vi "WS1050 36 DUT Reliability HD_Cycling Ver1.5a.vi"() -> ()   [LabVIEW 2012]
uses:
  WS_VCAP Driver 029/Source/WSVCAP Shell/Type Defs/WSVCAP SHL I2C DUT Mask Mode Enum.ctl
  <vilib>/Utility/file.llb/Read From Spreadsheet File (DBL).vi
panel:
  out "VISA resource name out":refnum<visa-resource-name>="GPIB0::3::INSTR"
  out "error out 2":errorcluster={"status"=TRUE, "code"=-63192, "source"="niLvFpga_Open_PXI-7813R.vi"}
  in  "Reg1_Bit Cntrl":string[](array[string])=["01", "02", "04", "08", "10", "20", "40", "80", "03", "06", "0C", "D8", "33", "66", "CC", "07", "0E", "1C", "38", "70", "E0", "0F", "1E", "3C", "78", "F0", "1F", "3E", "7C", "F8", "3F", "7E", "FC", "7F", "FE", "FD", "FB", "F7", "EF", "DF", "BF", "7F", "FC", "F9", "F3", "E7", "CF", "9F", "3F", "F8", "F1", "E3", "C7", "8F", "1F", "F0", "E1", "C3", "87", "0F", "E0", "C1", "83", "07", "C0", "81", "03", "AA", "55", "00"]
  out "date string":string="5/19/2014"
  out "PS1 Out":refnum<visa-resource-name>
  out "Ke2000 Out":refnum<visa-resource-name>="GPIB0::9::INSTR"
  in  "VPI_Cmd":string[](array[string])=["00", "3B", "00"]
  in  "VPI Name":string[](array[string])=["All_Drivers OFF", "All Drivers ON", "All Drivers OFF2"]
  in  "Tab Control":T1(tab)
  in  "Board#":string="BRD5"
  in  "Serial Number":string[][](table)=[["DUT", "SN"], ["DUT1", "1"], ["DUT2", "2"], ["DUT3", "3"], ["DUT4", "4"], ["DUT5", "5"], ["DUT6", "6"], ["DUT7", "7"], ["DUT8", "8"], ["DUT9", "9"], ["DUT10", "10"], ["DUT11", "11"], ["DUT12", "12"], ["DUT13", "13"], ["DUT14", "14"], ["DUT15", "15"], ["DUT16", "16"], ["DUT17", "17"], ["DUT18", "18"], ["DUT19", "19"], ["DUT20", "20"], ["DUT21", "21"], ["DUT22", "22"], ["DUT23", "23"], ["DUT24", "24"], ["DUT25", "25"], ["DUT26", "26"], ["DUT27", "27"], ["DUT28", "28"], ["DUT29", "29"], ["DUT30", "30"], ["DUT31", "31"], ["DUT32", "32"], ["DUT33", "33"], ["DUT34", "34"], ["DUT35", "35"], ["DUT36", "36"]]
  in  "Wafer#":string="T7-EB"
  in  "File Name":string="CYC_WS1050_T7_EB_65C_40V_25DC_EMPTY_BRD5_151017_1"
  in  "TMN DC\\CAP Data Log File Path":path=path "C:/WS1050 36 DUT Data"
  in  "Test Program":string="WS1050 36 DUT Reliability HD_Cycling Ver1.5a"
  in  "Comment":string="CYC65C40V"
  in  "Calibration":bool
  out "AR  Measurent(Hz)":dbl
  in  "PS1 Source":refnum<visa-resource-name>="GPIB0::5::INSTR"
  in  "Ke2000":refnum<visa-resource-name>="GPIB0::9::INSTR"
  out "Simulate FPGA":bool
  out "Online":bool
  out "AR Cycling(Hz)":dbl=5000000.0
  in  "Ke2400":refnum<visa-resource-name>="GPIB0::3::INSTR"
  in  "Initialize AD7747":bool
  in  "DUT Mask Mode":T2=enum."All"
  in  "RFFE Slave Address":u8=7 caption="Slave Address" format="0x%02x"
  out "Activity Log":string="05/19/2014 -- 12:24:35.853::WSVCAP::APP::Application Started\n05/19/2014 -- 12:24:37.606::WSVCAP::WSVCAP SHL::WR I2C-REG:0x0A;MASK:0xFFFFFFFFFFFF;C1 DATA:22:22:22:22:22:22:22:22:22:22:22:22:22:22:22:22;C2 DATA:22:22:22:22:22:22:22:22:22:22:22:22:22:22:22:22;C3 DATA:22:22:22:22:22:22:22:22:22:22:22:22:22:22:22:22\r\n05/19/2014 -- 12:24:37.773::WSVCAP::WSVCAP SHL::WR I2C-ST:0,0,4,1\r\n05/19/2014 -- 12:24:37.903::WSVCAP::WSVCAP SHL::RD I2C-BYTES:4;ADD:0x00;MASK:0xFFFFFFFFFFFF\r\n05/19/2014 -- 12:24:38.045::WSVCAP::WSVCAP SHL::RD I2C:C1 DATA:2:2:2:2:2:2:2:2:2:2:2:2:2:2:2:2|A7:A9:AA:82:82:7F:82:81:82:81:83:82:81:82:82:81|46:36:BB:88:44:A3:E9:2B:32:20:ED:25:BB:3D:68:B|2C:6A:EB:A7:22:56:FE:CC:36:82:D7:B0:3B:48:F9:CC;C2 DATA:2:2:2:2:2:2:2:2:2:2:2:2:2:2:2:2|94:94:94:80:80:80:80:80:81:7E:7E:81:80:7E:80:80|47:33:15:82:62:B:E8:1C:D7:C3:7D:41:7C:B7:4C:2A|C4:B4:AE:8:1E:D1:4E:37:11:C0:6F:63:42:9D:63:B5;C3 DATA:2:2:2:2:2:2:2:2:2:2:2:2:2:2:2:2|95:95:95:81:81:7E:81:80:84:7D:80:83:81:7E:7F:80|AB:C4:14:B5:7B:52:DF:C9:79:5D:5F:30:99:31:1E:F4|6E:5C:F7:A8:C3:EB:7B:EF:33:92:89:77:4D:67:75:DD;STATUS:0:0:4:0\r\n05/19/2014 -- 12:24:38.046::WSVCAP::WSVCAP SHL::WR I2C-REG:0x0A;MASK:0xFFFFFFFFFFFF;C1 DATA:22:22:22:22:22:22:22:22:22:22:22:22:22:22:22:22;C2 DATA:22:22:22:22:22:22:22:22:22:22:22:22:22:22:22:22;C3 DATA:22:22:22:22:22:22:22:22:22:22:22:22:22:22:22:22\r\n05/19/2014 -- 12:24:38.089::WSVCAP::WSVCAP SHL::WR I2C-ST:0,0,4,1\r\n05/19/2014 -- 12:24:38.219::WSVCAP::WSVCAP SHL::RD I2C-BYTES:4;ADD:0x00;MASK:0xFFFFFFFFFFFF\r\n05/19/2014 -- 12:24:38.362::WSVCAP::WSVCAP SHL::RD I2C:C1 DATA:2:2:2:2:2:2:2:2:2:2:2:2:2:2:2:2|A7:AB:AA:82:82:82:83:83:82:82:82:82:7F:82:82:81|4B:32:96:83:3E:61:43:17:25:62:AB:4D:A2:40:2E:5|3C:76:2B:B4:EE:E4:A9:1A:AA:A:26:C7:21:2E:87:5B;C2 DATA:2:2:2:2:2:2:2:2:2:2:2:2:2:2:2:2|94:94:94:80:80:80:80:80:80:7F:80:81:80:80:7F:80|4A:32:19:7D:19:6C:79:46:61:7F:4B:B8:A5:30:F3:14|B4:70:A:8C:9C:DC:43:FA:1E:A:C6:21:A:A9:13:F3;C3 DATA:2:2:2:2:2:2:2:2:2:2:2:2:2:2:2:2|95:97:94:81:80:81:82:81:80:7E:81:84:7F:81:80:80|B2:32:D0:A7:9E:4C:AB:D4:EE:D9:F0:82:B7:91:7:FF|C1:91:B6:3D:D8:E:1B:4F:9F:6A:F1:6C:E7:3F:7:BA;STATUS:0:0:4:0\r\n05/19/2014 -- 12:24:38.364::WSVCAP::WSVCAP SHL::WR I2C-REG:0x0A;MASK:0xFFFFFFFFFFFF;C1 DATA:22:22:22:22:22:22:22:22:22:22:22:22:22:22:22:22;C2 DATA:22:22:22:22:22:22:22:22:22:22:22:22:22:22:22:22;C3 DATA:22:22:22:22:22:22:22:22:22:22:22:22:22:22:22:22\r\n05/19/2014 -- 12:24:38.406::WSVCAP::WSVCAP SHL::WR I2C-ST:0,0,4,1\r\n05/19/2014 -- 12:24:38.536::WSVCAP::WSVCAP SHL::RD I2C-BYTES:4;ADD:0x00;MASK:0xFFFFFFFFFFFF\r\n05/19/2014 -- 12:24:38.678::WSVCAP::WSVCAP SHL::RD I2C:C1 DATA:2:2:2:2:2:2:2:2:2:2:2:2:2:2:2:2|A7:A9:AB:82:82:81:82:82:82:82:82:82:82:82:82:81|46:71:4C:87:43:3D:7F:FC:25:4F:8E:54:97:3E:60:8C|AA:F4:1F:B5:CE:43:1F:36:9:87:9C:78:86:5:B6:8E;C2 DATA:2:2:2:2:2:2:2:2:2:2:2:2:2:2:2:2|94:94:94:80:7F:7F:80:80:80:80:80:81:80:80:80:80|49:36:18:7D:6E:C5:E4:3C:81:2E:41:D3:75:71:E3:72|E8:D3:E6:D1:E0:48:AE:D4:54:D:E8:8E:B4:41:68:4;C3 DATA:2:2:2:2:2:2:2:2:2:2:2:2:2:2:2:2|95:95:95:81:7F:7F:81:81:81:81:81:84:81:81:82:81|B3:F5:90:AB:82:69:7B:93:D0:77:E8:D5:E8:8C:84:E8|B9:AC:EE:2B:B6:71:8F:4A:74:31:56:BB:8A:B7:A0:C8;STATUS:0:0:4:0\r\n05/19/2014 -- 12:24:38.681::WSVCAP::WSVCAP SHL::WR I2C-REG:0x0A;MASK:0xFFFFFFFFFFFF;C1 DATA:22:22:22:22:22:22:22:22:22:22:22:22:22:22:22:22;C2 DATA:22:22:22:22:22:22:22:22:22:22:22:22:22:22:22:22;C3 DATA:22:22:22:22:22:22:22:22:22:22:22:22:22:22:22:22\r\n05/19/2014 -- 12:24:38.723::WSVCAP::WSVCAP SHL::WR I2C-ST:0,0,4,1\r\n05/19/2014 -- 12:24:38.854::WSVCAP::WSVCAP SHL::RD I2C-BYTES:4;ADD:0x00;MASK:0xFFFFFFFFFFFF\r\n05/19/2014 -- 12:24:38.996::WSVCAP::WSVCAP SHL::RD I2C:C1 DATA:2:2:2:2:2:2:2:2:2:2:2:2:2:2:2:2|A7:A9:AA:82:82:7F:83:81:82:81:84:82:7F:82:7F:82|43:FB:E:7F:3C:AD:35:35:26:A2:6C:21:4B:3D:8:6|63:9A:E1:F3:95:32:91:42:90:3C:78:1F:5C:D7:5F:D8;C2 DATA:2:2:2:2:2:2:2:2:2:2:2:2:2:2:2:2|94:94:94:80:80:80:80:80:81:80:7E:81:80:7E:7F:80|48:36:18:7F:5E:3D:69:83:DE:AE:A1:9E:31:AE:BB:96|15:A0:44:17:13:FD:CC:C8:6D:B2:EF:A7:C:C7:3B:F;C3 DATA:2:2:2:2:2:2:2:2:2:2:2:2:2:2:2:2|95:96:94:81:81:7E:82:80:84:80:80:84:7F:7E:7D:82|AD:3B:6D:A9:7C:57:9D:F5:7A:96:23:5C:36:2D:ED:5A|CD:46:DB:3B:C7:BD:70:60:33:B8:B:F7:63:A:51:4D;STATUS:0:0:4:0\r\n05/19/2014 -- 12:24:38.998::WSVCAP::WSVCAP SHL::WR I2C-REG:0x0A;MASK:0xFFFFFFFFFFFF;C1 DATA:22:22:22:22:22:22:22:22:22:22:22:22:22:22:22:22;C2 DATA:22:22:22:22:22:22:22:22:22:22:22:22:22:22:22:22;C3 DATA:22:22:22:22:22:22:22:22:22:22:22:22:22:22:22:22\r\n05/19/2014 -- 12:24:39.040::WSVCAP::WSVCAP SHL::WR I2C-ST:0,0,4,1\r\n05/19/2014 -- 12:24:39.170::WSVCAP::WSVCAP SHL::RD I2C-BYTES:4;ADD:0x00;MASK:0xFFFFFFFFFFFF\r\n05/19/2014 -- 12:24:39.311::WSVCAP::WSVCAP SHL::RD I2C:C1 DATA:2:2:2:2:2:2:2:2:2:2:2:2:2:2:2:2|A7:AA:AB:82:82:81:82:81:82:81:82:82:82:82:7F:82|44:F1:90:87:45:44:C8:2C:2C:F1:FC:1B:94:3B:3C:75|4A:49:95:19:99:73:64:3:23:24:F3:A2:5E:7F:C4:B6;C2 DATA:2:2:2:2:2:2:2:2:2:2:2:2:2:2:2:2|94:94:94:80:80:80:80:7F:80:80:7E:80:80:7E:7F:80|4C:36:17:7D:A8:9F:DE:C7:53:6D:8A:F4:41:A5:C6:E0|90:2E:24:C:D9:22:E4:76:3B:40:1D:53:33:B1:3E:4D;C3 DATA:2:2:2:2:2:2:2:2:2:2:2:2:2:2:2:2|95:97:95:81:81:7F:81:80:80:81:7F:82:81:7E:7D:82|AE:2B:A7:AB:CC:CD:A4:38:FD:17:80:F2:92:2D:45:C4|76:E5:D:B9:AD:B5:BA:8D:28:32:9E:42:B7:20:4A:D9;STATUS:0:0:4:0\r\n05/19/2014 -- 12:24:39.313::WSVCAP::WSVCAP SHL::WR I2C-REG:0x0A;MASK:0xFFFFFFFFFFFF;C1 DATA:22:22:22:22:22:22:22:22:22:22:22:22:22:22:22:22;C2 DATA:22:22:22:22:22:22:22:22:22:22:22:22:22:22:22:22;C3 DATA:22:22:22:22:22:22:22:22:22:22:22:22:22:22:22:22\r\n05/19/2014 -- 12:24:39.355::WSVCAP::WSVCAP SHL::WR I2C-ST:0,0,4,1\r\n05/19/2014 -- 12:24:39.486::WSVCAP::WSVCAP SHL::RD I2C-BYTES:4;ADD:0x00;MASK:0xFFFFFFFFFFFF\r\n05/19/2014 -- 12:24:39.628::WSVCAP::WSVCAP SHL::RD I2C:C1 DATA:2:2:2:2:2:2:2:2:2:2:2:2:2:2:2:2|A7:A9:AA:82:82:82:83:82:82:82:82:82:7F:82:7F:82|47:18:E4:87:3E:E7:6:65:25:92:37:38:A8:3E:89:85|7C:A7:7:2B:A3:7A:EC:EF:89:ED:F4:D3:D8:BC:3A:F5;C2 DATA:2:2:2:2:2:2:2:2:2:2:2:2:2:2:2:2|94:94:94:80:7F:80:80:7F:81:80:7E:80:80:80:81:80|49:37:17:80:76:25:6A:F8:DF:55:97:4D:B8:5B:2B:B1|13:E3:9A:3E:1A:2D:4F:B6:DB:E9:61:FA:8B:D6:9:CC;C3 DATA:2:2:2:2:2:2:2:2:2:2:2:2:2:2:2:2|95:95:95:81:7F:80:82:81:84:80:7F:81:80:81:7F:82|AF:93:3B:AF:5B:11:82:E4:7E:C3:2D:72:9:96:D9:A|DB:96:F2:10:5F:64:9A:C6:98:12:27:7D:10:D3:20:D9;STATUS:0:0:4:0\r\n05/19/2014 -- 12:24:40.132::WSVCAP::WSVCAP SHL::CLOSE\r\n"
  in  "C1 Cap DAC":u8=128 caption="B Data In" format="0x%02x"
  in  "C2 Cap DAC":u8=128 caption="B Data In" format="0x%02x"
  in  "C3 Cap DAC":u8=128 caption="B Data In" format="0x%02x"
  in  "Lot#":string="WS1050"
  out "AD7747 Values":string[][](table)
  in  "SPI Clock Rate (Hz)":dbl=5000000.0 caption="Cycle Speed" format="%.1p Hz"
  in  "Clock Rate (Hz)":dbl=1000000.0 caption="Meas Speed" format="%.1p Hz"
  in  "Tab Control 2":enum32{"CPV", "Setup Stress", "Start Run"}(tab)
  in  "CP VPI":i32(ring) items=["CP HDC 35V", "CP HDC 40.25V", "CP HDC 27.5V", "CP HDC 30.5V", "CP HDC 44V", "CP HDC 50V", "CP HDC 55V", "CP HDC 42.5V", "CP HDC 32V"]
  in  "CP to Meas":i32(ring)=1 items=["CP HDC 35V", "CP HDC 40.25V", "CP HDC 27.5V", "CP HDC 30.5V", "CP HDC 44V", "CP HDC 50V", "CP HDC 55V", "CP HDC 42.5V", "CP HDC 32V"]
  in  "CP to HD/Cycle":i32(ring)=1 items=["CP HDC 35V", "CP HDC 40.25V", "CP HDC 27.5V", "CP HDC 30.5V", "CP HDC 44V", "CP HDC 50V", "CP HDC 55V", "CP HDC 42.5V", "CP HDC 32V"]
  in  "CP with DVA ON":i32(ring) items=["CP HDC 35V", "CP HDC 40.25V", "CP HDC 27.5V", "CP HDC 30.5V", "CP HDC 44V", "CP HDC 50V", "CP HDC 55V", "CP HDC 42.5V", "CP HDC 32V"]
  in  "CP Setting":i32(ring) items=["CP OFF", "CP ON", "CP 35V", "CP 40V", "DVA ON", "DVA OFF", "REG1 ON", "REG1 OFF", "REG2 ON", "REG2 OFF", "REG3 ON", "REG3 OFF"]
  in  "Verify CP":bool
  in  "Set VDD":dbl=3.7 format="%.3g"
  in  "Reset P/S":bool
  out "IDD Brd(uA)":string
  out "IDD Stdby(uA)":string="2.606990E+0"
  out "NOM IDD ON (uA)":string
  out "NOM IDD OFF(uA)":string
  out "IDD_HD/CYC (uA)":string="164.601255E+0"
  out "HS":bool
  out "VSA":bool
  out "VPI":bool
  out "DVA":bool
  out "E-CAL":bool
  out "HD/CYC":bool
  out "Verify Socket":bool
  in  "Control Panel":T3={"Verify Socket"=FALSE, "HD/CYC"=FALSE, "E-CAL"=FALSE, "DVA"=FALSE, "VPI"=TRUE, "VSA"=TRUE, "HS"=TRUE}
  in  "Post CMd Delay":dbl[](array[numeric])=[1.7e-05, 5.4e-05, 1.8e-05] min=0.0 max=0.5 format="%#.0p s"
  in  "% Duty Cycle":string="25"
  in  "Command":string[](array[string])=["0702013B3B3B", "070201000000", "0702013B0000"]
  in  "No of Cmd":i64=2
  in  "Cmd To HD":string="0702013B3B3B"
  in  "Freq(Hz)":string="12K"
  in  "Repeat Meas(s)":u32=300
  in  "Real No. From\nLookup Table":bool
  out "Cmd for Special Stress":string[](array[string])
  in  "Cmin/Act":bool=TRUE
  in  "Accumulative Stress":bool
  in  "Select Cycles Seq":u16(ring) items=["L_MSB", "M_LSB", "L_M_LSB", "M_L_MSB"]
  in  "OK Button":bool
  in  "Start Time":string="1542"
  in  "Start Date":string="10/21/2014"
  out "Current Time":string="0950"
  out "Current Date":string="8/28/2014"
  out "error out":errorcluster
  in  "error in (no error)":errorcluster
  in  "WS1050/51":bool=TRUE
  in  "Test Sequences":i32(ring) items=["C1_C2_C3", "C2_C1_C3", "C3_C2_C1"]
  out "CAP_C1":string[][](table)
  out "CAP_C2":string[][](table)
  out "CAP_C3":string[][](table)
  out "Total Time":u64
  in  "Set Stress run":u64=5000000000
  out "Completed Stress":u64
  out "Cycle Count":u64 min=1 max=4 step=1
  out "Loop \ncompleted":i32=1
  out "Previous Time":string="12:20:26 PM"
  out "STATUS":string="Idle...."
  out "Total Delta C2(pF)":string[](array[string])
  out "Total Delta C1(pF)":string[](array[string])
  out "Total Delta C3(pF)":string[](array[string])
  out "RB Reg for HD":string[](array[string])
  out "RB Reg for HD/Cycle":string[](array[string])
  out "VPI C2":string[][](table)
  out "VPI C3":string[][](table)
  in  "stop During HD/Cycles":bool
  in  "stop":bool
  out "VPI C1":string[][](table)
  out "VSA_V1":string[][](table)
  out "VSA_V2":string[][](table)
  out "VSA_V3":string[][](table)
  in  "VSA Voltage(V)":dbl[](array[numeric])=[-10.0, 0.0, 10.0]
  in  "DC_Temp":i32=65
  in  "HD/CYC Temp":i32=65
  in  "Time All ON (s)":u32=120
  in  "Time All OFF (s)":u32=120
  in  "HD_DC (Min)":u64=259200
  out "LPs Count":i32
  in  "X Repeat":i32=100
  out "No LPs to RP":i32
  out "Run Loops":i32=1
  out "TTCompleted":u64=2000
  in  "TTF Completed":u64=5000000000
  out "% Delta C_T0":string[][](array[string])
  out "% Delta C":string[][](array[string])
  out "EFuse RB T0":string[](array[string])
  out "Current EFuse Read back":string[](array[string])
  out "EFuse Readback Status":bool[](array[boolean])
  in  "DeltaC Target Setting(pF)":dbl=7.375
  in  "HD RP":dbl=60.0
  in  "Cycle RP":dbl=10000.0
  in  "Bank C3":i32(ring)=2 items=["C1", "C2", "C3", "D_C1", "D_C2", "D_C3"]
  in  "Bank C2":i32(ring)=1 items=["C1", "C2", "C3", "D_C1", "D_C2", "D_C3"]
  in  "Bank C1":i32(ring) items=["C1", "C2", "C3", "D_C1", "D_C2", "D_C3"]
  out "Min Plot_1":dbl[][](graph) caption="(Y) Multi Plot 2"
  out "Min Plot_2":dbl[][](graph) caption="(Y) Multi Plot 2"
  out "Min Plot_3":dbl[][](graph) caption="(Y) Multi Plot 2"
  in  "Debug":bool
  in  "No of Rows\nFrom Spread Sheet":i32
  in  "Plot Delta Cmin":bool=TRUE
  in  "Plot":T4(ring)
  # "Company:  WiSpry Inc\n20 Fairbanks Ste 198 \nIrvine CA 92618\n\nAuthor:  Andy V Tran\nCreated:  02/15/2016\nLabVIEW 2012 Pro\nTest Program:  WS1050 36 DUT Reliability HD_Cycling ver1.5a\nFPGA: WS_VCAP Driver 029"
  # "Note for HD Duty Cycle:\n1.  Set time to start HD_DC (Min), = 6 or 24 hrs; default is 259200 (6 months) \n2.  Set Time for HD_CYC ON/OFF, default setting is 2 Min ON + 2 Min OFF with specific time.  Normally is 48hrs.\n3.  Set HD/Cycle to completed = item 1 + item 2 = 6 or 24hrs + 48 hrs\n4.  Set X Repeat = number of runs, default is 100 runs; each run is = item 3\n5.  Set TTF Completed to stop the test.\n\nVer 1.5 updated based on Ver1.4:\n1.  Updated calibration procedure by changing offset cal in series"
  # "Minutes"
  # "X1000"
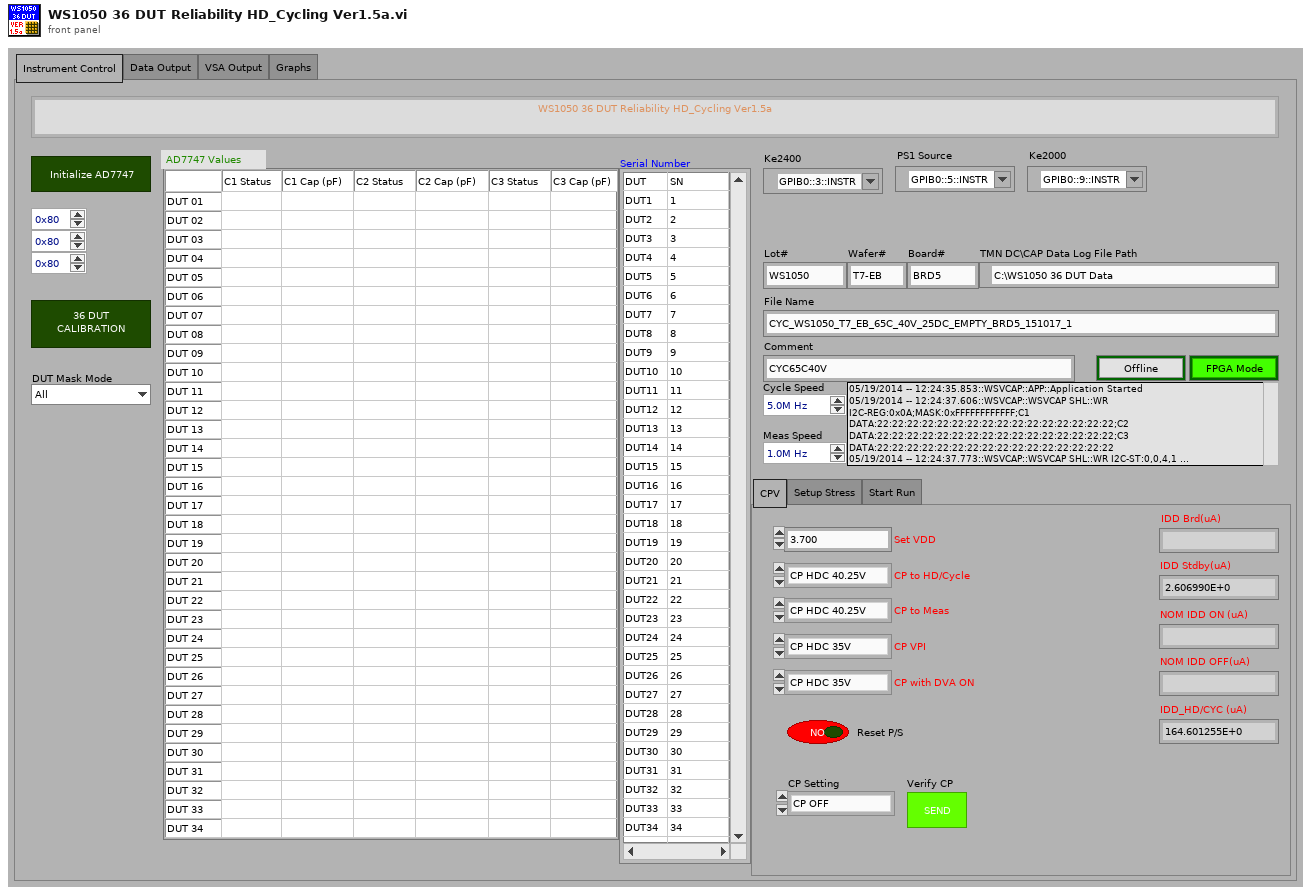
[diagram p1: front panel]
types:
  T1 = enum32{"Instrument Control", "Data Output", "VSA Output", "Graphs"}
  T2 = typedef "WSVCAP SHL I2C DUT Mask Mode Enum.ctl" = enum16{"Custom", "C1", "C2", "C3", "All"}
  T3 = cluster{"Verify Socket":bool, "HD/CYC":bool, "E-CAL":bool, "DVA":bool, "VPI":bool, "VSA":bool, "HS":bool}
  T4 = enum16{"ALL DUTs", "DUT 01", "DUT 02", "DUT 03", "DUT 04", "DUT 05", "DUT 06", "DUT 07", "DUT 08", "DUT 09", "DUT 10", "DUT 11", "DUT 12", "DUT 13", "DUT 14", "DUT 15", "DUT 16", "DUT 17", "DUT 18", "DUT 19", "DUT 20", "DUT 21", "DUT 22", "DUT 23", "DUT 24", "DUT 25", "DUT 26", "DUT 27", "DUT 28", "DUT 29", "DUT 30", "DUT 31", "DUT 32", "DUT 33", "DUT 34", "DUT 35", "DUT 36"}
  T5 = typedef "WSVCAP SHL Core System Cluster.ctl" = cluster{"Settings":T6, "FPGA Resource":tag, "Online":bool, "I2C Wait Ticks":u32, "SPI Wait Ticks":u32, "RFFE Wait Ticks":u32}
  T6 = typedef "WSVCAP SHL I2C Settings Cluster.ctl" = cluster{"FPGA Resource Name":string, "I2C Slave Address":u8, "I2C Clock Rate (Hz)":dbl, "SPI Clock Rate (Hz)":dbl, "RFFE Slave Address":u8, "RFFE Clock Rate (Hz)":dbl, "Simulate FPGA":bool, "C1 Cap DAC Default":u8, "C2 Cap DAC Default":u8, "C3 Cap DAC Default":u8}
  T7 = enum16{"Idle...", "Voltage 1", "Voltage 2", "Voltage 3"}[]
  T8 = cluster{"Test Program ":string, "Comment":string, "Data Out":string, "Data Out":string, "Data Out":string, string, "Data Out":string, "Data Out":string, "Data Out":string, "Freq(Hz)":string, "Board#":string}
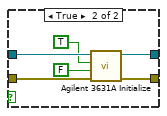
[diagram p2: hidden frame]
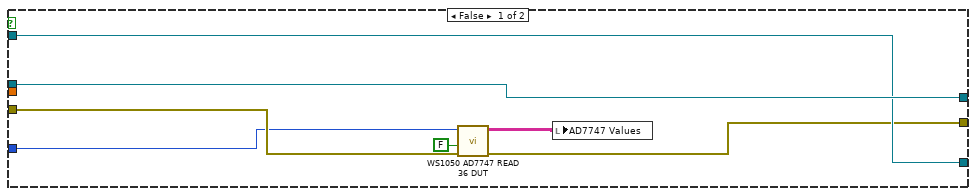
[diagram p10: hidden frame]
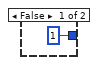
[diagram p11: hidden frame]
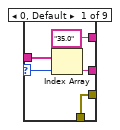
[diagram p12: hidden frame]
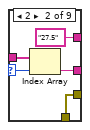
[diagram p13: hidden frame]
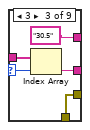
[diagram p14: hidden frame]
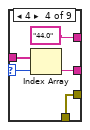
[diagram p15: hidden frame]
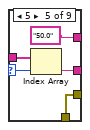
[diagram p16: hidden frame]
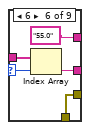
[diagram p17: hidden frame]
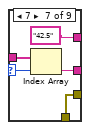
[diagram p18: hidden frame]
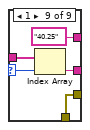
[diagram p19: hidden frame]
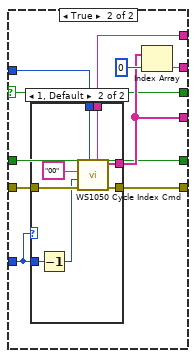
[diagram p20: hidden frame]
diagram:
  w25 = TRUE
  w29 = u16 0 items=["Off", "Moving Filter", "Repeating Filter"] ("Digital Filter (0: Off)")
  w30 = u16 7 items=["3.5 Digits"=4, "4.5 Digits"=5, "5.5 Digits"=6, "6.5 Digits"=7] ("Resolution (7: 6.5 digits)")
  n1 = case shown="True" w25 {
    tunnel: "error in (no error)" -> [w37 w38]
    tunnel: [w37 w45] -> w14
    frame False {
    }
    frame True {
      n2 = call "WSVCAP SHL Host TL Initialize.vi"("error in"=w38) -> ("error out"=w39:errorcluster)  [unwired: 13 in, 1 out]
      n3 = control-ref of="Activity Log"() -> (w41:refnum<vi>)
      n4 = call "ACT LG Activity Log Core.vi"("Display Ref"=w41, "Source"="WSVCAP", "Error In (no error)"=w39) -> ("Error Out"=w40:errorcluster)  [unwired: 11 in, 1 out]
      n5 = call "WSVCAP SHL Host TL Status Manager.vi"("error in"=w40) -> ("System Out"=w46:T5, "error out"=w45:errorcluster)  [unwired: 13 in]
      n6 = Unbundle By Name(w46) -> ("Online"=→"Online":bool, "Settings.Simulate FPGA"=→"Simulate FPGA":bool)
    }
  }
  n7 = case shown="True" TRUE {
    tunnel: w14 -> [w47 w52]
    tunnel: [w48 w51] -> w22
    tunnel: [w47 w50] -> w18
    tunnel: "Ke2400" -> [w48 w49]
    frame False {
    }
    frame True {
      n8 = VISA Write(VISA resource name=w49, write buffer="SOUR:FUNC VOLT;VOLT:MODE FIX;RANG 100;LEV 0.0;:SENS:FUNC \"CURR\";CURR:PROT 60E-3;RANG 100E-3;:OUTP ON", error in (no error)=w52) -> (VISA resource name out=w51:refnum<visa-resource-name>, error out=w50:errorcluster)  [unwired: 1 out]
    }
  }
  n9 = case shown="False" "Reset P/S" {
    tunnel: "PS1 Source" -> [w54 w61]
    tunnel: [w54 w59] -> w34
    tunnel: w14 -> [w55 w57]
    tunnel: [w55 w56] -> w13
    frame False {
    }
    frame True {
      n10 = call "Agilent 3631A Initialize.vi"("error in (no error)"=w57, "Default"=FALSE ("Reset? (T: Yes)"), "Reset"=TRUE ("ID Query? (T: Yes)"), "VISA resource name"=w61) -> ("error out"=w56:errorcluster, "VISA resource name out"=w59:refnum<visa-resource-name>)  [unwired: 6 in]
    }
  }
  n11 = call "Ke2000 Initialize.vi"("error in (no error)"=w14, "VISA resource name"="Ke2000") -> ("error out"=w31:errorcluster, "VISA resource name out"=w32:refnum<visa-resource-name>)  [unwired: 8 in]
  n12 = call "Ke2000 Configure DC Current.vi"("Resolution (7: 6.5 digits)"=w30, "Digital Filter (0: Off)"=w29, "Auto Range? (T: Auto)"=FALSE, "error in"=w31, "Custom Range (0 A)"=1.0, "VISA resource name"=w32) -> ("error out"=w15:errorcluster, "VISA resource name out"=w27:refnum<visa-resource-name>)  [unwired: 4 in]
  n13 = case shown="True" TRUE {
    tunnel: [_ w62] -> w36
    frame False {
    }
    frame True {
      n14 = call-poly <vilib>:"Read From Spreadsheet File.vi"("number of rows (all:-1)"=-1) -> ("all rows"=w62:dbl[][])  [unwired: 6 in, 4 out]
    }
  }
  n15 = Merge Errors(w18, w15, w13) -> (w23:errorcluster)
  n16 = while {
    tunnel: w23 -> [w70]
    tunnel: [w66] -> w4
    tunnel: w36 -> [w93]
    tunnel: w34 -> [w81]
    tunnel: w27 -> [w82]
    tunnel: [w91] -> w10
    tunnel: [w90] -> w5
    tunnel: w22 -> [w88]
    tunnel: [w87] -> w20
    tunnel: [FALSE ("stop")] -> w16
    i -> [w89]
    stop <- w94 stop-if-true
    n17 = case shown="0" w89 {
      tunnel: w70 -> [w104 w106]
      tunnel: [w103 w106] -> w84
      tunnel: "RFFE Slave Address" -> [w101 _]
      frame 0 {
        w97 = dbl[][] []
        w96 = "" ("uA")
        w98 = string[][] []
        w99 = string[] [] ("EFuse Read back")
        w105 = u64 0 ("No of HD/Cycle\nCompleted")
        n18 = local write "RB Reg for HD/Cycle"(w99) -> ()
        n19 = local write "Current EFuse Read back"(w99) -> ()
        n20 = local write "EFuse RB T0"(w99) -> ()
        n21 = local write "Total Delta C1(pF)"(w99) -> ()
        n22 = local write "Total Delta C2(pF)"(w99) -> ()
        n23 = local write "Total Delta C3(pF)"(w99) -> ()
        n24 = local write "Cycle Count"(w105) -> ()
        n25 = local write "Completed Stress"(w105) -> ()
        n26 = local write "CAP_C2"(w98) -> ()
        n27 = local write "CAP_C1"(w98) -> ()
        n28 = local write "VPI C2"(w98) -> ()
        n29 = local write "VSA_V3"(w98) -> ()
        n30 = local write "VSA_V1"(w98) -> ()
        n31 = local write "NOM IDD OFF(uA)"(w96) -> ()
        n32 = local write "NOM IDD ON (uA)"(w96) -> ()
        n33 = local write "IDD Brd(uA)"(w96) -> ()
        n34 = local write "VSA_V2"(w98) -> ()
        n35 = local write "CAP_C3"(w98) -> ()
        n36 = local write "VPI C1"(w98) -> ()
        n37 = local write "VPI C3"(w98) -> ()
        n38 = local write "% Delta C"(w98) -> ()
        n39 = local write "% Delta C_T0"(w98) -> ()
        n40 = call "WSVCAP SHL Host TL RFFE Configure.vi"("RFFE Slave Address"=w101, "Clock Rate (Hz)"="Clock Rate (Hz)", "error in"=w104) -> ("Actual Rate (Hz)"=→"AR  Measurent(Hz)":dbl, "error out"=w103:errorcluster)  [unwired: 11 in]
        n41 = local write "Min Plot_3"(w97) -> ()
        n42 = local write "Min Plot_1"(w97) -> ()
        n43 = local write "Min Plot_2"(w97) -> ()
      }
      frame 1, Default {
      }
    }
    n44 = while {
      tunnel: ["stop"] -> w86
      tunnel: w84 -> [w137]
      tunnel: [w130] -> w78
      tunnel: w81 -> [w136]
      tunnel: w82 -> [w132]
      tunnel: [w133] -> w80
      tunnel: [w131] -> w79
      tunnel: [w128] -> w77
      tunnel: [w127] -> w76
      tunnel: [w126] -> w75
      tunnel: [w125] -> w74
      tunnel: [w124] -> w73
      tunnel: [w123] -> w72
      tunnel: [w122] -> w71
      tunnel: ["Command"] -> w69
      tunnel: ["Post CMd Delay"] -> w68
      tunnel: "Set VDD" -> [w112]
      stop <- w144 stop-if-true
      # "Set Date & Time to Start Test"
      n45 = case shown="True" "Initialize AD7747" {
        tunnel: w137 -> [w153 w159]
        tunnel: [w153 w155] -> w121
        tunnel: w136 -> [w152 w157]
        tunnel: [w152 w156] -> w135
        tunnel: w112 -> [_ w154]
        frame False {
        }
        frame True {
          w160 = T7 [enum."Voltage 2", enum."Voltage 3", enum."Voltage 1"] items=["Idle...", "Voltage 1", "Voltage 2", "Voltage 3"]
          n46 = for {
            tunnel: w157 -> [w170]
            tunnel: w160 -> [w168] mode=indexing
            tunnel: [w167] -> w156
            shift-right: [w164] -> w158
            shift-left: w159 -> [w171]
            tunnel: w154 -> [w161]
            n47 = call "E3631A_Voltage Controller updated.vi"("VISA resource name"=w170, "I_VDD(A)"=0.5, "Channel Controller"=w168, "Voltage 1"=w161, "Voltage 2"=3.3, "error in (no error)"=w171, "I_3.3V (A)"=0.5) -> ("VISA resource name out"=w167:refnum<visa-resource-name>, "error out"=w163:errorcluster)  [unwired: 7 in]
            n48 = call "Delay.vi"("milliseconds to wait"=u32 100, "error in (no error)"=w163) -> ("error out"=w164:errorcluster)  [unwired: 9 in]
          }
          n49 = call "WS1050_AD7747_Init 36DUT.vi"("error in"=w158) -> ("error out"=w155:errorcluster)  [unwired: 10 in]
        }
      }
      n50 = call "Time_stamp.vi"() -> ("date/time string"=w149:string, "date string"=w151:string)  [unwired: 2 in]
      "Current Date" <- w151
      "Current Time" <- w149
      n51 = Equal?(x=w151, y="Start Date") -> (x = y?=w147:bool)
      n52 = Equal?(x=w149, y="Start Time") -> (x = y?=w146:bool)
      n53 = And(x=w147, y=w146) -> (x .and. y?=w143:bool)
      n54 = Compound Arithmetic op=OR(w143, "OK Button", "stop") -> (w144:bool)
      n55 = case shown="True" "Calibration" {
        tunnel: w121 -> [w201 w219]
        tunnel: [w197 w216] -> w119
        tunnel: w135 -> [w200 w215]
        tunnel: [w200 w212] -> w134
        tunnel: w132 -> [w199 w211]
        tunnel: [w199 w208] -> w131
        tunnel: w112 -> [_ w207]
        tunnel: "DUT Mask Mode" -> [w196 w205]
        tunnel: "C1 Cap DAC" -> [_ w204]
        tunnel: "C2 Cap DAC" -> [_ w203]
        tunnel: "C3 Cap DAC" -> [_ w202]
        frame False {
          n56 = call "WS1050 AD7747 READ 36 DUT.vi"("error in"=w201, "Log (T)"=FALSE, "DUT Mask Mode (All)"=w196) -> ("error out"=w197:errorcluster, "AD7747 Values"=w195:string[][])  [unwired: 7 in]
          n57 = local write "AD7747 Values"(w195) -> ()
        }
        frame True {
          n58 = flat-sequence {
            tunnel: w219 -> [w221]
            tunnel: [w227] -> w218
            tunnel: w215 -> [w230]
            tunnel: [w229] -> w214
            tunnel: w211 -> [w226]
            tunnel: [w225] -> w210
            tunnel: w207 -> [w224]
            tunnel: [w223] -> w206
            tunnel: w205 -> [w223]
            tunnel: w218 -> [w255]
            tunnel: [w244] -> w217
            tunnel: w214 -> [w257]
            tunnel: [w257] -> w213
            tunnel: w210 -> [w256]
            tunnel: [w256] -> w209
            tunnel: w206 -> [w243]
            tunnel: w204 -> [w252]
            tunnel: w203 -> [w251]
            tunnel: w202 -> [w250]
            tunnel: w217 -> [w259]
            tunnel: [w258] -> w216
            tunnel: w213 -> [w263]
            tunnel: [w261] -> w212
            tunnel: w209 -> [w260]
            tunnel: [w260] -> w208
            frame #0 {
              w231 = T7 [enum."Voltage 2", enum."Voltage 3", enum."Voltage 1"] items=["Idle...", "Voltage 1", "Voltage 2", "Voltage 3"]
              n59 = for {
                tunnel: w230 -> [w242]
                tunnel: w231 -> [w240] mode=indexing
                tunnel: [w239] -> w229
                tunnel: w224 -> [w234]
                tunnel: w221 -> [w233]
                tunnel: [w232] -> w220
                n60 = call "E3631A_Voltage Controller updated.vi"("VISA resource name"=w242, "I_VDD(A)"=0.5, "Channel Controller"=w240, "Voltage 1"=w234, "Voltage 2"=3.3, "error in (no error)"=w233, "I_3.3V (A)"=0.5) -> ("VISA resource name out"=w239:refnum<visa-resource-name>, "error out"=w237:errorcluster)  [unwired: 7 in]
                n61 = call "Delay.vi"("milliseconds to wait"=u32 100, "error in (no error)"=w237) -> ("error out"=w232:errorcluster)  [unwired: 9 in]
              }
              n62 = call "Ke2000 Single Reading.vi"("error in (no error)"=w220, "VISA resource name"=w226) -> ("error out"=w227:errorcluster, "VISA resource name out"=w225:refnum<visa-resource-name>, "uA"=→"IDD Brd(uA)":string)  [unwired: 5 in, 2 out]
              n63 = One Button Dialog(message="Please verify all sockets should be empty...") -> ()  [unwired: 1 in, 1 out]
            }
            frame #1 {
              n64 = call "WS1050 CAPDAC Setting Updated.vi"("DUT Mask Mode (All)"=w243, "error in"=w255, "C3 Cap DAC"=w250, "C2 Cap DAC"=w251, "C1 Cap DAC"=w252) -> ("error out"=w253:errorcluster)  [unwired: 6 in]
              n65 = call "WS1050 OFFSET CAL updated.vi"("error in"=w253, "OFFSET CAL"=TRUE ("Read?")) -> ("error out"=w248:errorcluster)  [unwired: 9 in]
              n66 = call "Delay.vi"("milliseconds to wait"=u32 100, "error in (no error)"=w248) -> ("error out"=w247:errorcluster)  [unwired: 9 in]
              n67 = call "WS1050 AD7747 READ 36 DUT.vi"("error in"=w247, "Log (T)"=FALSE, "DUT Mask Mode (All)"=w243) -> ("error out"=w244:errorcluster, "AD7747 Values"=→"AD7747 Values":string[][])  [unwired: 7 in]
            }
            frame #2 {
              w262 = T7 [enum."Voltage 2", enum."Voltage 3", enum."Voltage 1"] items=["Idle...", "Voltage 1", "Voltage 2", "Voltage 3"]
              n68 = for {
                tunnel: w263 -> [w274]
                tunnel: w262 -> [w272] mode=indexing
                tunnel: [w271] -> w261
                tunnel: w259 -> [w266]
                tunnel: [w265] -> w258
                w267 = 0.5 ("I_VDD(A)")
                n69 = call "E3631A_Voltage Controller updated.vi"("VISA resource name"=w274, "I_VDD(A)"=w267, "Channel Controller"=w272, "Voltage 1"=0.0, "Voltage 2"=3.3, "error in (no error)"=w266, "I_3.3V (A)"=w267) -> ("VISA resource name out"=w271:refnum<visa-resource-name>, "error out"=w268:errorcluster)  [unwired: 7 in]
                n70 = call "Delay.vi"("milliseconds to wait"=u32 100, "error in (no error)"=w268) -> ("error out"=w265:errorcluster)  [unwired: 9 in]
              }
              n71 = One Button Dialog(message="Calibration Completed....") -> ()  [unwired: 1 in, 1 out]
            }
          }
        }
      }
      n72 = local write "stop During HD/Cycles"(FALSE ("stop During HD/Cycles")) -> ()
      n73 = call "Control Panel.vi"("error in (no error)"=w121, "Control Panel"="Control Panel") -> ("error out"=w118:errorcluster, "VPI"=w124:bool, "DVA"=w125:bool, "E-CAL"=w126:bool, "VSA"=w123:bool, "HD/CYC"=w127:bool, "HS"=w122:bool, "Verify Socket"=w128:bool)  [unwired: 2 in]
      "Verify Socket" <- w128
      "E-CAL" <- w126
      "VPI" <- w124
      "VSA" <- w123
      "HS" <- w122
      "HD/CYC" <- w127
      "DVA" <- w125
      n74 = Merge Errors(w118, w119) -> (w120:errorcluster)
      n75 = case shown="True" "Verify CP" {
        tunnel: [w172 w178] -> w130
        tunnel: w134 -> [w173 w180]
        tunnel: [w173 w179] -> w133
        tunnel: w120 -> [w172 w175]
        tunnel: w112 -> [_ w176]
        frame False {
        }
        frame True {
          w181 = T7 [enum."Voltage 2", enum."Voltage 3", enum."Voltage 1"] items=["Idle...", "Voltage 1", "Voltage 2", "Voltage 3"]
          # "Verify CP"
          n76 = for {
            tunnel: w180 -> [w194]
            tunnel: w181 -> [w192] mode=indexing
            tunnel: [w189] -> w179
            tunnel: w176 -> [w188]
            tunnel: w175 -> [w186]
            tunnel: [w185] -> w174
            w187 = 0.5 ("I_VDD(A)")
            n77 = call "E3631A_Voltage Controller updated.vi"("VISA resource name"=w194, "I_VDD(A)"=w187, "Channel Controller"=w192, "Voltage 1"=w188, "Voltage 2"=3.3, "error in (no error)"=w186, "I_3.3V (A)"=w187) -> ("VISA resource name out"=w189:refnum<visa-resource-name>, "error out"=w191:errorcluster)  [unwired: 7 in]
            n78 = call "Delay.vi"("milliseconds to wait"=u32 100, "error in (no error)"=w191) -> ("error out"=w185:errorcluster)  [unwired: 9 in]
          }
          n79 = Index Array(array=string[] ["074000", "074040", "07476F", "074776", "074800", "074820", "07413B", "074100", "07423B", "074200", "07433B", "074300"], index="CP Setting") -> (element=w182:string)
          n80 = call "WSVCAP SHL Host TL RFFE Write - Multiple DUTs - Common Data.vi"("Data Out"=w182, "error in"=w174, "Log (T)"=FALSE) -> ("error out"=w178:errorcluster)  [unwired: 12 in]
        }
      }
      n81 = Array Subset(array="Post CMd Delay", length="No of Cmd") -> (w116:dbl[])  [unwired: 1 in]
      n82 = Array Subset(array="Command", length="No of Cmd") -> (w117:string[])  [unwired: 1 in]
      n83 = property on="Post CMd Delay" class="Arr (strict)"("Number of Rows"="No of Cmd") -> ()  [unwired: 2 in, 2 out]
      n84 = local write "Command"(w117) -> ()
      n85 = local write "Post CMd Delay"(w116) -> ()
      n86 = property on="Command" class="Arr (strict)"("Number of Rows"="No of Cmd") -> ()  [unwired: 2 in, 2 out]
      n87 = Wait Until Next ms Multiple(millisecond multiple=u32 100) -> ()  [unwired: 1 out]
    }
    n88 = case shown="False" w86 {
      tunnel: w78 -> [w337 w1980]
      tunnel: [w322 w1980] -> w66
      tunnel: w93 -> [w338 _]
      tunnel: w80 -> [w336 w1978]
      tunnel: w79 -> [w328 w1979]
      tunnel: [w334 w1979] -> w91
      tunnel: [w332 w1978] -> w90
      tunnel: w88 -> [w325 w1977]
      tunnel: [w321 w1977] -> w87
      tunnel: "RFFE Slave Address" -> [w316 _]
      tunnel: w77 -> [w297 _]
      tunnel: w76 -> [w296 _]
      tunnel: w75 -> [w279 _]
      tunnel: w74 -> [w295 _]
      tunnel: w73 -> [w294 _]
      tunnel: w72 -> [w293 _]
      tunnel: w71 -> [w292 _]
      tunnel: w69 -> [w286 _]
      tunnel: w68 -> [w285 _]
      tunnel: "Set VDD" -> [w284 _]
      tunnel: [w281 FALSE ("stop During HD/Cycles")] -> w64
      frame False {
        w317 = u64 0 ("Total Completed")
        w302 = u32 100 ("milliseconds to wait")
        w333 = T7 [enum."Voltage 2", enum."Voltage 3", enum."Voltage 1"] items=["Idle...", "Voltage 1", "Voltage 2", "Voltage 3"]
        w335 = T7 [enum."Voltage 2", enum."Voltage 3", enum."Voltage 1"] items=["Idle...", "Voltage 1", "Voltage 2", "Voltage 3"]
        # "E-CAL ON/OFF"
        n89 = for {
          tunnel: w337 -> [w1975]
          tunnel: w336 -> [w1974]
          tunnel: w335 -> [w1972] mode=indexing
          tunnel: [w1968] -> w330
          tunnel: [w1971] -> w320
          tunnel: w284 -> [w1965]
          n90 = call "E3631A_Voltage Controller updated.vi"("VISA resource name"=w1974, "I_VDD(A)"=0.5, "Channel Controller"=w1972, "Voltage 1"=w1965, "Voltage 2"=3.3, "error in (no error)"=w1975, "I_3.3V (A)"=0.5) -> ("VISA resource name out"=w1971:refnum<visa-resource-name>, "error out"=w1969:errorcluster)  [unwired: 7 in]
          n91 = call "Delay.vi"("milliseconds to wait"=u32 100, "error in (no error)"=w1969) -> ("error out"=w1968:errorcluster)  [unwired: 9 in]
        }
        n92 = local write "TTCompleted"(w317) -> ()
        n93 = local write "Total Time"(w317) -> ()
        n94 = call "WSVCAP SHL Host TL RFFE Write - Multiple DUTs - Common Data.vi"("Data Out"="074000", "error in"=w330, "Log (T)"=FALSE) -> ("error out"=w331:errorcluster)  [unwired: 12 in]
        n95 = local read "IDD Brd(uA)"() -> (w305:string)
        n96 = call "Delay.vi"("milliseconds to wait"=w302, "error in (no error)"=w331) -> ("error out"=w329:errorcluster)  [unwired: 9 in]
        n97 = call "Ke2000 Single Reading.vi"("error in (no error)"=w329, "VISA resource name"=w328) -> ("error out"=w306:errorcluster, "VISA resource name out"=w327:refnum<visa-resource-name>, "uA"=w308:string)  [unwired: 5 in, 2 out]
        n98 = for {
          N: 36 -> [_]
          tunnel: "Serial Number" -> [w347]
          tunnel: [w345] -> w299 mode=indexing
          i -> [w344]
          n99 = Increment(x=w344) -> (x+1=w343:i32)
          n100 = Index Array(array=w347, index (row)=w343, index (col)=1 ("disabled index (col)")) -> (element=w345:string)
        }
        n101 = call "Substration.vi"("error in (no error)"=w306, "Input2"=w305, "Input1"=w308) -> ("error out"=w288:errorcluster, "In1 - In2"=w307:string)  [unwired: 7 in]
        "IDD Stdby(uA)" <- w307
        n102 = Number To Fractional String(number=w284, precision (6)=i16 2) -> (F-format string=w310:string)  [unwired: 2 in]
        n103 = case shown="True" w296 {
          tunnel: [1 ("X Repeat") w349] -> w319
          frame False {
          }
          frame True {
            n104 = local read "X Repeat"() -> (w349:i32)
          }
        }
        n105 = call "WSVCAP SHL Host TL RFFE Write - Multiple DUTs - Common Data.vi"("Data Out"="074040", "error in"=w288, "Log (T)"=FALSE) -> ("error out"=w287:errorcluster)  [unwired: 12 in]
        n106 = call "Delay.vi"("milliseconds to wait"=w302, "error in (no error)"=w287) -> ("error out"=w314:errorcluster)  [unwired: 9 in]
        n107 = call "WS1050 DVA CP Setting.vi"("error in (no error)"=w314, "DVA"=w295, "CP with DVA ON"="CP with DVA ON") -> ("error out"=w312:errorcluster, "Data Out"=w313:string)  [unwired: 7 in]
        n108 = call "Delay.vi"("milliseconds to wait"=w302, "error in (no error)"=w312) -> ("error out"=w278:errorcluster)  [unwired: 9 in]
        n109 = Not(x=w292) -> (.not. x?=w298:bool)
        n110 = call "WS1050 ECAL.vi"("error in (no error)"=w278, "E-CAL"=w279) -> ("error out"=w277:errorcluster, "Data Out"=w276:string)  [unwired: 8 in]
        n111 = for {
          N: w319 -> [_]
          tunnel: w338 -> [w387]
          tunnel: [w383] -> w334
          tunnel: w307 -> [w382]
          tunnel: w327 -> [w381]
          tunnel: "TMN DC\\CAP Data Log File Path" -> [w380]
          tunnel: w325 -> [w378]
          tunnel: [w377] -> w323
          tunnel: w320 -> [w354]
          shift-right: [w372] -> _
          shift-left: u64 0 -> [w374]
          tunnel: w296 -> [w371]
          tunnel: w316 -> [w366]
          tunnel: w316 -> [w365]
          tunnel: w313 -> [w364]
          tunnel: w310 -> [w363]
          tunnel: [w362] -> w304
          tunnel: w277 -> [w361]
          tunnel: w295 -> [w360]
          tunnel: w297 -> [w359]
          tunnel: w294 -> [w358]
          tunnel: w298 -> [w357]
          tunnel: w293 -> [w356]
          tunnel: w299 -> [w355]
          tunnel: [w354] -> w289
          tunnel: w286 -> [w353]
          tunnel: w285 -> [w352]
          tunnel: [w351] -> w280
          tunnel: w276 -> [w350]
          i -> [w370]
          stop <- w351 stop-if-true
          n112 = while {
            tunnel: w387 -> [w611]
            tunnel: w380 -> [w622]
            tunnel: "Lot#" -> [w621]
            tunnel: "Wafer#" -> [w620]
            tunnel: w355 -> [w619]
            tunnel: "Test Program" -> [w618]
            tunnel: w355 -> [w617]
            tunnel: "Comment" -> [w616]
            tunnel: "Lot#" -> [w615]
            tunnel: "Wafer#" -> [w614]
            tunnel: w381 -> [w610]
            tunnel: [w613] -> w383
            tunnel: w382 -> [w609]
            tunnel: w378 -> [w606]
            tunnel: [w605] -> w377
            tunnel: [w513] -> w368
            tunnel: w370 -> [w551]
            tunnel: [w542] -> w372
            tunnel: w374 -> [w541]
            shift-right: [w540] -> _
            shift-left: u64 0 -> [w439]
            tunnel: [w539] -> w367
            tunnel: w371 -> [w537]
            tunnel: w366 -> [w512]
            tunnel: w365 -> [w510]
            tunnel: w364 -> [w460]
            tunnel: w363 -> [w458]
            tunnel: [w436] -> w362
            tunnel: w361 -> [w392]
            tunnel: w360 -> [w441]
            tunnel: w359 -> [w433]
            tunnel: w358 -> [w432]
            tunnel: w357 -> [w427]
            tunnel: w356 -> [w421]
            tunnel: w353 -> [w397]
            tunnel: w352 -> [w396]
            tunnel: w350 -> [w391]
            i -> [w538]
            stop <- w552 stop-if-true
            n113 = case shown="8" "CP to HD/Cycle" {
              selector: "CP to HD/Cycle" -> [w626 w631 w636 w641 w646 w651 w656 w661 w665]
              tunnel: string[] ["07476F", "074776", "074765", "074769", "07477B", "07477C", "07477D", "074779", "07476B"] -> [w627 w632 w637 w642 w647 w652 w657 w662 w667]
              tunnel: [w625 w630 w635 w640 w645 w650 w655 w660 w666] -> w456
              tunnel: ["35.0" ("Data Out") "27.5" ("Data Out") "30.5" ("Data Out") "44.0" ("Data Out") "50.0" ("Data Out") "55.0" ("Data Out") "42.5" ("Data Out") "32.0" ("Data Out") "40.25" ("Data Out")] -> w455
              tunnel: [w623 w628 w633 w638 w643 w648 w653 w658 w663] -> w454
              tunnel: w392 -> [w623 w628 w633 w638 w643 w648 w653 w658 w663]
              frame 0, Default {
                n114 = Index Array(array=w627, index=w626) -> (element=w625:string)
              }
              frame 2 {
                n115 = Index Array(array=w632, index=w631) -> (element=w630:string)
              }
              frame 3 {
                n116 = Index Array(array=w637, index=w636) -> (element=w635:string)
              }
              frame 4 {
                n117 = Index Array(array=w642, index=w641) -> (element=w640:string)
              }
              frame 5 {
                n118 = Index Array(array=w647, index=w646) -> (element=w645:string)
              }
              frame 6 {
                n119 = Index Array(array=w652, index=w651) -> (element=w650:string)
              }
              frame 7 {
                n120 = Index Array(array=w657, index=w656) -> (element=w655:string)
              }
              frame 8 {
                n121 = Index Array(array=w662, index=w661) -> (element=w660:string)
              }
              frame 1 {
                n122 = Index Array(array=w667, index=w665) -> (element=w666:string)
              }
            }
            n123 = flat-sequence {
              tunnel: [w744] -> w604
              tunnel: [w739] -> w603
              tunnel: w611 -> [w742]
              tunnel: [w741] -> w602
              tunnel: w610 -> [w720]
              tunnel: w609 -> [w740]
              tunnel: [w740] -> w601
              tunnel: [w699] -> w600
              tunnel: [w696] -> w599
              tunnel: w454 -> [w732]
              tunnel: w551 -> [w737]
              tunnel: w538 -> [w669]
              tunnel: [w669] -> w548
              tunnel: w538 -> [w736]
              tunnel: w537 -> [w734]
              tunnel: [w733] -> w536
              tunnel: [w704] -> w531
              tunnel: [w703] -> w530
              tunnel: [w702] -> w529
              tunnel: [w708] -> w519
              tunnel: [w705] -> w518
              tunnel: w512 -> [w731]
              tunnel: [w731] -> w511
              tunnel: w510 -> [w730]
              tunnel: [w707] -> w498
              tunnel: [w706] -> w473
              tunnel: [w729] -> w461
              tunnel: w456 -> [w727]
              tunnel: [w719] -> w453
              tunnel: [w690] -> w445
              tunnel: w433 -> [w718]
              tunnel: w432 -> [w717]
              tunnel: [w717] -> w431
              tunnel: w427 -> [w716]
              tunnel: [w716] -> w426
              tunnel: w421 -> [w715]
              tunnel: [w715] -> w420
              tunnel: [w711] -> w415
              tunnel: ["Test Sequences"] -> w411
              tunnel: "Real No. From\nLookup Table" -> [w671]
              tunnel: ["WS1050/51"] -> w405
              tunnel: ["Cmin/Act"] -> w401
              tunnel: w397 -> [w682]
              tunnel: w396 -> [w691]
              tunnel: "Accumulative Stress" -> [w680]
              tunnel: "Select Cycles Seq" -> [w679]
              tunnel: [w676] -> w388
              tunnel: w604 -> [w1072]
              tunnel: w603 -> [w1097]
              tunnel: w602 -> [w1102]
              tunnel: [w1102] -> w509
              tunnel: w601 -> [w1101]
              tunnel: w600 -> [w1096]
              tunnel: w599 -> [w1095]
              tunnel: [w1086] -> w508
              tunnel: [w1101] -> w507
              tunnel: [w1096] -> w506
              tunnel: [w1095] -> w505
              tunnel: w548 -> [w1099]
              tunnel: [w1099] -> w504
              tunnel: w536 -> [w1098]
              tunnel: [w1098] -> w503
              tunnel: [w1097] -> w502
              tunnel: w531 -> [w1094]
              tunnel: w530 -> [w1079]
              tunnel: w529 -> [w1080]
              tunnel: [w1091] -> w501
              tunnel: w519 -> [w1093]
              tunnel: w518 -> [w1091]
              tunnel: [w1087] -> w500
              tunnel: w511 -> [w1092]
              tunnel: [w1077] -> w499
              tunnel: w498 -> [w1077]
              tunnel: [w1079] -> w497
              tunnel: w473 -> [w1078]
              tunnel: [w1078] -> w472
              tunnel: [w1080] -> w470
              tunnel: w461 -> [w1090]
              tunnel: [w1089] -> w446
              tunnel: w445 -> [w1089]
              tunnel: w431 -> [w1085]
              tunnel: [w1085] -> w430
              tunnel: w426 -> [w1084]
              tunnel: [w1084] -> w425
              tunnel: w420 -> [w1083]
              tunnel: [w1083] -> w419
              tunnel: w415 -> [w1082]
              tunnel: [w1081] -> w414
              tunnel: w411 -> [w1075]
              tunnel: [w1075] -> w410
              tunnel: w405 -> [w1074]
              tunnel: [w1074] -> w404
              tunnel: w401 -> [w1073]
              tunnel: [w1073] -> w400
              tunnel: [w1072] -> w394
              tunnel: w509 -> [w1224]
              tunnel: [w1224] -> w494
              tunnel: w508 -> [w1206]
              tunnel: [w1206] -> w492
              tunnel: w507 -> [w1223]
              tunnel: [w1223] -> w490
              tunnel: w506 -> [w1222]
              tunnel: [w1222] -> w488
              tunnel: w505 -> [w1221]
              tunnel: [w1221] -> w486
              tunnel: w504 -> [w1220]
              tunnel: [w1220] -> w484
              tunnel: w503 -> [w1219]
              tunnel: [w1219] -> w482
              tunnel: w502 -> [w1218]
              tunnel: [w1218] -> w480
              tunnel: w501 -> [w1217]
              tunnel: [w1217] -> w478
              tunnel: [w1211] -> w476
              tunnel: w500 -> [w1210]
              tunnel: w499 -> [w1215]
              tunnel: w497 -> [w1214]
              tunnel: w472 -> [w1203]
              tunnel: [w1203] -> w471
              tunnel: w470 -> [w1205]
              tunnel: [w1205] -> w469
              tunnel: [w1212] -> w468
              tunnel: [w1213] -> w447
              tunnel: w446 -> [w1213]
              tunnel: w430 -> [w1209]
              tunnel: [w1209] -> w429
              tunnel: w425 -> [w1208]
              tunnel: [w1208] -> w424
              tunnel: w419 -> [w1207]
              tunnel: [w1207] -> w418
              tunnel: w414 -> [w1204]
              tunnel: w410 -> [w1201]
              tunnel: [w1204] -> w409
              tunnel: [w1201] -> w408
              tunnel: w404 -> [w1200]
              tunnel: [w1200] -> w403
              tunnel: w400 -> [w1199]
              tunnel: [w1199] -> w399
              tunnel: w394 -> [w1198]
              tunnel: [w1198] -> w393
              tunnel: [w1291] -> w496
              tunnel: [w1303] -> w495
              tunnel: w494 -> [w1318]
              tunnel: [w1318] -> w493
              tunnel: w492 -> [w1297]
              tunnel: [w1297] -> w491
              tunnel: w490 -> [w1317]
              tunnel: [w1317] -> w489
              tunnel: w488 -> [w1316]
              tunnel: [w1316] -> w487
              tunnel: w486 -> [w1315]
              tunnel: [w1315] -> w485
              tunnel: w484 -> [w1314]
              tunnel: [w1314] -> w483
              tunnel: w482 -> [w1313]
              tunnel: [w1313] -> w481
              tunnel: w480 -> [w1312]
              tunnel: [w1312] -> w479
              tunnel: w478 -> [w1311]
              tunnel: [w1311] -> w477
              tunnel: w476 -> [w1310]
              tunnel: [w1310] -> w475
              tunnel: [w1294] -> w474
              tunnel: w471 -> [w1308]
              tunnel: w469 -> [w1307]
              tunnel: w468 -> [w1302]
              tunnel: ["DeltaC Target Setting(pF)"] -> w459
              tunnel: [w1305] -> w448
              tunnel: w447 -> [w1305]
              tunnel: w441 -> [w1304]
              tunnel: [w1304] -> w440
              tunnel: w429 -> [w1301]
              tunnel: [w1301] -> w428
              tunnel: w424 -> [w1300]
              tunnel: [w1300] -> w423
              tunnel: w418 -> [w1299]
              tunnel: [w1299] -> w417
              tunnel: w409 -> [w1298]
              tunnel: w408 -> [w1295]
              tunnel: [w1294] -> w406
              tunnel: w403 -> [w1293]
              tunnel: [w1293] -> w402
              tunnel: w399 -> [w1292]
              tunnel: [w1292] -> w398
              tunnel: w393 -> [w1291]
              tunnel: [w1385] -> w598
              tunnel: [w1405] -> w597
              tunnel: w496 -> [w1385]
              tunnel: w495 -> [w1419]
              tunnel: [w1428] -> w596
              tunnel: [w1419] -> w595
              tunnel: [w1441] -> w594
              tunnel: [w1440] -> w593
              tunnel: w493 -> [w1439]
              tunnel: [w1439] -> w592
              tunnel: w491 -> [w1428]
              tunnel: w489 -> [w1438]
              tunnel: [w1438] -> w591
              tunnel: w487 -> [w1434]
              tunnel: [w1434] -> w590
              tunnel: w485 -> [w1433]
              tunnel: [w1433] -> w589
              tunnel: w483 -> [w1429]
              tunnel: [w1429] -> w547
              tunnel: w481 -> [w1437]
              tunnel: [w1437] -> w535
              tunnel: w479 -> [w1436]
              tunnel: [w1435] -> w532
              tunnel: w477 -> [w1431]
              tunnel: w475 -> [w1427]
              tunnel: [w1432] -> w528
              tunnel: [w1430] -> w527
              tunnel: [w1427] -> w522
              tunnel: w474 -> [w1426]
              tunnel: [w1413] -> w517
              tunnel: [w1412] -> w516
              tunnel: [w1411] -> w515
              tunnel: w459 -> [w1425]
              tunnel: [w1410] -> w449
              tunnel: w448 -> [w1410]
              tunnel: [w1409] -> w444
              tunnel: w440 -> [w1408]
              tunnel: w428 -> [w1403]
              tunnel: w423 -> [w1402]
              tunnel: [w1402] -> w422
              tunnel: w417 -> [w1401]
              tunnel: [w1401] -> w416
              tunnel: w406 -> [w1398]
              tunnel: w402 -> [w1397]
              tunnel: w398 -> [w1386]
              tunnel: w598 -> [w1636]
              tunnel: [w1636] -> w588
              tunnel: [w1663] -> w587
              tunnel: [w1677] -> w586
              tunnel: w597 -> [w1676]
              tunnel: w596 -> [w1675]
              tunnel: w595 -> [w1674]
              tunnel: [w1675] -> w585
              tunnel: [w1674] -> w584
              tunnel: w594 -> [w1673]
              tunnel: [w1673] -> w583
              tunnel: w593 -> [w1672]
              tunnel: [w1672] -> w582
              tunnel: w592 -> [w1671]
              tunnel: [w1671] -> w581
              tunnel: w591 -> [w1670]
              tunnel: [w1670] -> w580
              tunnel: w590 -> [w1669]
              tunnel: [w1669] -> w579
              tunnel: w589 -> [w1668]
              tunnel: [w1668] -> w578
              tunnel: w606 -> [w1667]
              tunnel: [w1665] -> w577
              tunnel: [w1645] -> w576
              tunnel: [w1646] -> w575
              tunnel: [w1644] -> w574
              tunnel: w547 -> [w1661]
              tunnel: [w1661] -> w546
              tunnel: w535 -> [w1660]
              tunnel: [w1660] -> w534
              tunnel: w532 -> [w1677]
              tunnel: w528 -> [w1658]
              tunnel: w527 -> [w1659]
              tunnel: [w1659] -> w526
              tunnel: [w1658] -> w524
              tunnel: w522 -> [w1657]
              tunnel: [w1657] -> w521
              tunnel: w517 -> [w1643]
              tunnel: w516 -> [w1642]
              tunnel: w515 -> [w1641]
              tunnel: [w1638] -> w514
              tunnel: [w1643] -> w467
              tunnel: [w1642] -> w465
              tunnel: [w1641] -> w463
              tunnel: [w1640] -> w450
              tunnel: w449 -> [w1640]
              tunnel: w444 -> [w1639]
              tunnel: [w1639] -> w443
              tunnel: w422 -> [w1638]
              tunnel: w416 -> [w1637]
              tunnel: w588 -> [w1785]
              tunnel: [w1785] -> w573
              tunnel: w587 -> [w1809]
              tunnel: [w1808] -> w572
              tunnel: w622 -> [w1810]
              tunnel: w621 -> [w1807]
              tunnel: w620 -> [w1806]
              tunnel: w619 -> [w1805]
              tunnel: [w1804] -> w571
              tunnel: w586 -> [w1798]
              tunnel: [w1798] -> w570
              tunnel: w585 -> [w1803]
              tunnel: w584 -> [w1802]
              tunnel: [w1803] -> w569
              tunnel: [w1802] -> w568
              tunnel: [w1793] -> w567
              tunnel: w583 -> [w1801]
              tunnel: [w1801] -> w566
              tunnel: w582 -> [w1800]
              tunnel: [w1800] -> w565
              tunnel: w581 -> [w1797]
              tunnel: [w1799] -> w564
              tunnel: w439 -> [w1796]
              tunnel: [w1795] -> w563
              tunnel: [w1783] -> w562
              tunnel: w580 -> [w1794]
              tunnel: w579 -> [w1792]
              tunnel: w578 -> [w1791]
              tunnel: "File Name" -> [w1790]
              tunnel: w577 -> [w1789]
              tunnel: [w1789] -> w561
              tunnel: w576 -> [w1788]
              tunnel: [w1788] -> w560
              tunnel: [w1787] -> w559
              tunnel: w575 -> [w1787]
              tunnel: w574 -> [w1786]
              tunnel: [w1786] -> w558
              tunnel: [w1781] -> w549
              tunnel: w546 -> [w1782]
              tunnel: [w1782] -> w544
              tunnel: w541 -> [w1780]
              tunnel: w534 -> [w1779]
              tunnel: [w1779] -> w533
              tunnel: w526 -> [w1778]
              tunnel: [w1778] -> w525
              tunnel: w524 -> [w1777]
              tunnel: [w1777] -> w523
              tunnel: w521 -> [w1776]
              tunnel: [w1776] -> w520
              tunnel: w514 -> [w1775]
              tunnel: w467 -> [w1774]
              tunnel: [w1774] -> w466
              tunnel: w465 -> [w1773]
              tunnel: [w1773] -> w464
              tunnel: w463 -> [w1772]
              tunnel: [w1772] -> w462
              tunnel: w453 -> [w1771]
              tunnel: [w1771] -> w452
              tunnel: [w1770] -> w451
              tunnel: w450 -> [w1770]
              tunnel: w443 -> [w1769]
              tunnel: [w1769] -> w442
              tunnel: ["Freq(Hz)"] -> w413
              tunnel: ["Board#"] -> w412
              tunnel: w573 -> [w1832]
              tunnel: w572 -> [w1883]
              tunnel: w622 -> [w1847]
              tunnel: w618 -> [w1878]
              tunnel: w617 -> [w1881]
              tunnel: w616 -> [w1877]
              tunnel: w615 -> [w1880]
              tunnel: w614 -> [w1876]
              tunnel: w571 -> [w1879]
              tunnel: [w1832] -> w554
              tunnel: [w1882] -> w555
              tunnel: w570 -> [w1875]
              tunnel: [w1875] -> w556
              tunnel: w569 -> [w1874]
              tunnel: w568 -> [w1859]
              tunnel: w567 -> [w1873]
              tunnel: w566 -> [w1872]
              tunnel: w565 -> [w1861]
              tunnel: [w1869] -> w557
              tunnel: w564 -> [w1871]
              tunnel: w563 -> [w1870]
              tunnel: w562 -> [w1869]
              tunnel: "File Name" -> [w1840]
              tunnel: w561 -> [w1868]
              tunnel: [w1868] -> w553
              tunnel: w560 -> [w1867]
              tunnel: w559 -> [w1866]
              tunnel: w558 -> [w1865]
              tunnel: [w1864] -> w550
              tunnel: w549 -> [w1864]
              tunnel: [w1843] -> w545
              tunnel: w544 -> [w1843]
              tunnel: w533 -> [w1863]
              tunnel: w525 -> [w1862]
              tunnel: w523 -> [w1860]
              tunnel: w520 -> [w1858]
              tunnel: w466 -> [w1857]
              tunnel: w464 -> [w1856]
              tunnel: w462 -> [w1855]
              tunnel: w460 -> [w1854]
              tunnel: w391 -> [w1853]
              tunnel: w455 -> [w1852]
              tunnel: w458 -> [w1851]
              tunnel: w452 -> [w1850]
              tunnel: w451 -> [w1849]
              tunnel: w442 -> [w1848]
              tunnel: [w1845] -> w438
              tunnel: [w1836] -> w434
              tunnel: w413 -> [w1835]
              tunnel: w412 -> [w1833]
              tunnel: w388 -> [w1830]
              tunnel: [w1934] -> w612
              tunnel: [w1935] -> w613
              tunnel: [w1936] -> w513
              tunnel: w557 -> [w1927]
              tunnel: w556 -> [w1935]
              tunnel: w555 -> [w1923]
              tunnel: w554 -> [w1936]
              tunnel: w553 -> [w1929]
              tunnel: [w1929] -> w605
              tunnel: [w1926] -> w542
              tunnel: w550 -> [w1926]
              tunnel: w545 -> [w1928]
              tunnel: [w1928] -> w543
              tunnel: [w1927] -> w540
              tunnel: [w1925] -> w539
              tunnel: [w1922] -> w435
              tunnel: w438 -> [w1921]
              tunnel: w434 -> [w1919]
              frame #0 {
                w712 = FALSE ("Log (T)")
                n124 = Index Array(array=w742, index (row)=w736, index (col)=0 ("disabled index (col)")) -> (element=w735:dbl)
                n125 = call "WSVCAP SHL Host TL RFFE Write - Multiple DUTs - Common Data.vi"("Data Out"=w727, "error in"=w732, "Log (T)"=FALSE) -> ("error out"=w675:errorcluster)  [unwired: 12 in]
                n126 = call "WS1050 Stress RB REG.vi"("error in (no error)"=w675, "Set RB REG"=string[] ["0760", "0767", "0768"]) -> ("error out"=w673:errorcluster, "Data out"=→"RB Reg for HD/Cycle":string[])  [unwired: 8 in]
                n127 = local read "IDD Brd(uA)"() -> (w726:string)
                n128 = call "Delay.vi"("milliseconds to wait"=u32 100, "error in (no error)"=w673) -> ("error out"=w722:errorcluster)  [unwired: 9 in]
                n129 = call "Ke2000 Single Reading.vi"("error in (no error)"=w722, "VISA resource name"=w720) -> ("error out"=w724:errorcluster, "VISA resource name out"=w701:refnum<visa-resource-name>, "uA"=w725:string)  [unwired: 5 in, 2 out]
                n130 = call "Substration.vi"("error in (no error)"=w724, "Input2"=w726, "Input1"=w725) -> ("error out"=w684:errorcluster, "In1 - In2"=→"IDD_HD/CYC (uA)":string)  [unwired: 7 in]
                n131 = case shown="False" w680 {
                  selector: w680 -> [w745 w753]
                  tunnel: w684 -> [w749 w761]
                  tunnel: [w748 w760] -> w683
                  tunnel: w682 -> [w747 _]
                  tunnel: [w747 w756] -> w681
                  tunnel: w679 -> [_ w759]
                  tunnel: ["Cmd To HD" w757] -> w678
                  tunnel: [w746 w755] -> w677
                  tunnel: w671 -> [w750 w752]
                  tunnel: [w750 w752] -> w670
                  tunnel: w669 -> [_ w754]
                  tunnel: [w745 w753] -> w668
                  frame False {
                    n132 = call "WS105x Stress Beams.vi"("error in (no error)"=w749, "Cycling Bit"=w747) -> ("error out"=w748:errorcluster, "Beams"=w746:string)  [unwired: 7 in, 1 out]
                  }
                  frame True {
                    n133 = case shown="1, Default" w754 {
                      tunnel: w761 -> [w764 w771]
                      tunnel: [w764 w770] -> w760
                      tunnel: w759 -> [_ w769]
                      tunnel: [string[] ["070201000000", "070201000000"] ("Cmd To Cycles") w768] -> w756
                      tunnel: ["T0" ("Stress Beams") w767] -> w755
                      tunnel: w754 -> [_ w766]
                      frame 0 {
                      }
                      frame 1, Default {
                        n134 = Decrement(x=w766) -> (x-1=w765:i32)
                        n135 = call "WS1050 Cycle Index Cmd.vi"("Select Cycles Seq"=w769, "error in (no error)"=w771, "Index"=w765, "OFF"="00") -> ("error out"=w770:errorcluster, "Cmd To Cycles"=w768:string[], "Stress Beams"=w767:string)  [unwired: 3 in, 2 out]
                      }
                    }
                    n136 = Index Array(array=w756, index=0) -> (element=w757:string)
                  }
                }
                n137 = case shown="False" w734 {
                  tunnel: [w862 w978] -> w744
                  tunnel: [w863 w964] -> w688
                  tunnel: [w861 w979] -> w741
                  tunnel: w737 -> [_ w969]
                  tunnel: w735 -> [w855 w965]
                  tunnel: [w859 w966] -> w733
                  tunnel: w669 -> [w847 w962]
                  tunnel: w730 -> [w857 _]
                  tunnel: ["% Duty Cycle" "100" ("Data Out")] -> w719
                  tunnel: w718 -> [w845 _]
                  tunnel: w670 -> [w844 _]
                  tunnel: w691 -> [w838 _]
                  tunnel: w683 -> [w841 w949]
                  tunnel: w681 -> [w840 _]
                  tunnel: w678 -> [_ w948]
                  tunnel: w677 -> [w839 w947]
                  tunnel: [w839 w947] -> w676
                  tunnel: w668 -> [w837 w946]
                  frame False {
                    # "Cycles in 1s"
                    n138 = case shown="False" w837 {
                      tunnel: w855 -> [w870 w885]
                      tunnel: [w869 w884] -> w854
                      tunnel: [w868 w885] -> w853
                      tunnel: [w867 u64 1000 ("y")] -> w848
                      tunnel: w847 -> [w866 _]
                      tunnel: w844 -> [w865 _]
                      tunnel: w841 -> [w864 w884]
                      frame False {
                        n139 = case shown="False" w865 {
                          tunnel: w864 -> [w876 w881]
                          tunnel: w870 -> [w875 w882]
                          tunnel: [w874 w881] -> w869
                          tunnel: w866 -> [w873 _]
                          tunnel: [w872 w882] -> w868
                          tunnel: [u64 1000 ("y") u64 1 ("y")] -> w867
                          frame False {
                            n140 = case shown="8, Default" w873 {
                              tunnel: w875 -> [w878 _]
                              tunnel: [w878 "Cycle RP"] -> w872
                              tunnel: [w877 w879] -> w874
                              tunnel: w876 -> [w877 w879]
                              frame 0..7 {
                              }
                              frame 8, Default {
                              }
                            }
                          }
                          frame True {
                            # "Read real \nnumber\nfrom \nlookup \ntable"
                          }
                        }
                      }
                      frame True {
                      }
                    }
                    n141 = Array Max & Min(array=w838) -> (max value=w851:dbl)  [unwired: 3 out]
                    n142 = Divide(x=1.0, y=w851) -> (x/y=w850:dbl)
                    n143 = To Unsigned Quad Integer(1:w850) -> (0:w849:u64)
                    n144 = call "WSVCAP SHL Host TL RFFE Configure.vi"("RFFE Slave Address"=w857, "Clock Rate (Hz)"="SPI Clock Rate (Hz)", "error in"=w854) -> ("Actual Rate (Hz)"=→"AR Cycling(Hz)":dbl, "error out"=w843:errorcluster)  [unwired: 11 in]
                    n145 = Not(x=w845) -> (.not. x?=w846:bool)
                    n146 = case shown="True" w846 {
                      tunnel: [w888 w910] -> w863
                      tunnel: [w891 w909] -> w862
                      tunnel: [u64 1 w908] -> w861
                      tunnel: w843 -> [w889 w907]
                      tunnel: w853 -> [_ w906]
                      tunnel: w838 -> [_ w904]
                      tunnel: w849 -> [_ w903]
                      tunnel: w848 -> [_ w902]
                      tunnel: w847 -> [w887 _]
                      tunnel: w840 -> [_ w901]
                      frame False {
                        n147 = case shown="1, Default" w887 {
                          tunnel: w889 -> [w892 w894]
                          tunnel: [w892 w893] -> w888
                          frame 0 {
                          }
                          frame 1, Default {
                            n148 = flat-sequence {
                              tunnel: "Repeat Meas(s)" -> [w900]
                              tunnel: w894 -> [w897]
                              tunnel: [w897] -> w893
                              frame #0 {
                                n149 = Multiply(x=w900, y=u32 1000) -> (x*y=w899:u32)
                                n150 = Wait (ms)(milliseconds to wait=w899) -> ()  [unwired: 1 out]
                                n151 = local write "STATUS"("Verify Sockets waiting times..." ("STATUS")) -> ()
                              }
                            }
                          }
                        }
                        n152 = local read "stop During HD/Cycles"() -> (w891:bool)
                      }
                      frame True {
                        n153 = while {
                          tunnel: w906 -> [w930]
                          tunnel: [w917] -> w910
                          tunnel: [w922] -> w909
                          tunnel: w907 -> [w928]
                          tunnel: [w916] -> w908
                          tunnel: w901 -> [w927]
                          tunnel: w904 -> [w926]
                          tunnel: w903 -> [w913]
                          tunnel: w902 -> [w911]
                          i -> [w925]
                          stop <- w921 stop-if-true
                          # "At least 1 second before target"
                          # "Remaining Cycles"
                          # "Target Cycles"
                          # "Cycles in 1s"
                          n154 = case shown="0" w925 {
                            tunnel: [w938 w940] -> w919
                            tunnel: w928 -> [w939 w940]
                            tunnel: w927 -> [w937 _]
                            tunnel: w926 -> [w936 _]
                            frame 0 {
                              n155 = call "WSVCAP SHL Host TL RFFE Write Cycle - Multiple DUTs - Common Data.vi"("Data Out (Cycle Commands)"=w937, "Post Command Delay"=w936, "error in"=w939, "Log (T)"=FALSE) -> ("error out"=w938:errorcluster)  [unwired: 11 in]
                            }
                            frame 1, Default {
                            }
                          }
                          n156 = To Unsigned Quad Integer(1:w930) -> (0:w929:u64)
                          n157 = Multiply(x=w929, y=w911) -> (x*y=w916:u64)
                          n158 = call "WSVCAP SHL Host TL SPI_RFFE Query Cycle Count.vi"("error in"=w919) -> ("Cycle Count"=w915:u64, "error out"=w924:errorcluster)  [unwired: 13 in]
                          "Cycle Count" <- w915
                          n159 = Subtract(x=w916, y=w915) -> (x-y=w914:u64)
                          n160 = Greater Or Equal?(x=w915, y=w916) -> (x >= y?=w923:bool)
                          n161 = local read "stop During HD/Cycles"() -> (w922:bool)
                          n162 = Greater?(x=w914, y=w913) -> (0:w912:bool)
                          n163 = case shown="True" w923 {
                            tunnel: [w942 w945] -> w918
                            tunnel: w924 -> [w942 w944]
                            tunnel: [FALSE TRUE] -> w920
                            frame False {
                            }
                            frame True {
                              n164 = call "WSVCAP SHL Host TL SPI Stop Write Cycle.vi"("error in"=w944) -> ("error out"=w945:errorcluster)  [unwired: 14 in]
                            }
                          }
                          n165 = Or(x=w920, y=w922) -> (x .or. y?=w921:bool)
                          n166 = case shown="True" w912 {
                            tunnel: w918 -> [w931 w934]
                            tunnel: [w931 w933] -> w917
                            frame False {
                            }
                            frame True {
                              n167 = call "MISC Wait with Data Flow.vi"("Error In (no error)"=w934, "Wait Time (500ms)"=u32 50) -> ("Error Out"=w933:errorcluster)  [unwired: 7 in, 2 out]
                            }
                          }
                        }
                        n168 = local write "STATUS"("Parts are Cycling...." ("STATUS")) -> ()
                      }
                    }
                    n169 = local read "HD/CYC Temp"() -> (w858:i32)
                    n170 = Number To Engineering String(4:w858) -> (0:w859:string)  [unwired: 3 in]
                    "Cmd for Special Stress" <- w840
                  }
                  frame True {
                    n171 = case shown="True" w946 {
                      tunnel: w969 -> [w985 _]
                      tunnel: [w984 w997] -> w968
                      tunnel: w949 -> [w983 w998]
                      tunnel: [w982 w998] -> w967
                      tunnel: w965 -> [w981 w997]
                      tunnel: w962 -> [w980 _]
                      frame False {
                        n172 = case shown="1, Default" w985 {
                          tunnel: [w988 w995] -> w984
                          tunnel: w983 -> [w990 w996]
                          tunnel: [w989 w996] -> w982
                          tunnel: w981 -> [w987 _]
                          tunnel: w980 -> [w986 _]
                          frame 0 {
                            n173 = case shown="0..14" w986 {
                              tunnel: [w991 "HD RP"] -> w988
                              tunnel: w990 -> [w992 w993]
                              tunnel: [w992 w993] -> w989
                              tunnel: w987 -> [w991 _]
                              frame 0..14 {
                              }
                              frame 15, Default {
                              }
                            }
                          }
                          frame 1, Default {
                            n174 = local read "HD RP"() -> (w995:dbl)
                          }
                        }
                      }
                      frame True {
                      }
                    }
                    n175 = local read "Completed Stress"() -> (w970:u64)
                    n176 = call "WSVCAP SHL Host TL RFFE Write - Multiple DUTs - Common Data.vi"("Data Out"=w948, "error in"=w967, "Log (T)"=FALSE) -> ("error out"=w955:errorcluster)  [unwired: 12 in]
                    n177 = call "Delay.vi"("milliseconds to wait"=u32 50, "error in (no error)"=w955) -> ("error out"=w952:errorcluster)  [unwired: 9 in]
                    n178 = Greater?(x="HD_DC (Min)", y=w970) -> (0:w971:bool)
                    n179 = call "WS1050 Stress RB REG.vi"("error in (no error)"=w952, "Set RB REG"=string[] ["0761", "0762", "0763"]) -> ("error out"=w974:errorcluster, "Data out"=→"RB Reg for HD":string[])  [unwired: 8 in]
                    n180 = case shown="True" w971 {
                      tunnel: [_ w1009] -> w976
                      tunnel: [w1000 w1008] -> w975
                      tunnel: w974 -> [w1000 w1007]
                      tunnel: w968 -> [w999 w1006]
                      tunnel: [w999 w1006] -> w973
                      frame False {
                      }
                      frame True {
                        n181 = Multiply(x=1000.0, y=w1006) -> (x*y=w1004:dbl)
                        n182 = Multiply(x=60.0, y=w1004) -> (x*y=w1002:dbl)
                        n183 = local write "STATUS"("Parts are Holding Down..." ("STATUS")) -> ()
                        n184 = event shown="[0] Timeout" {
                          selector: _ -> [_ _]
                          dyn-events: _ -> [_ _]
                          timeout: w1002 -> [_ _]
                          tunnel: ["stop During HD/Cycles" TRUE ("stop During HD/Cycles")] -> w1009
                          tunnel: w1007 -> [w1010 w1012]
                          tunnel: [w1010 w1012] -> w1008
                          event Timeout {
                            n185 = event-data() -> ()  [unwired: 1 in, 2 out]
                          }
                          event "stop During HD/Cycles": Value Change {
                            n186 = event-data() -> ()  [unwired: 1 in, 2 out]
                          }
                        }
                      }
                    }
                    n187 = Greater Or Equal?(x=w970, y="HD_DC (Min)") -> (x >= y?=w977:bool)
                    n188 = To Unsigned Quad Integer(1:w968) -> (0:w979:u64)
                    n189 = Add(x="Time All OFF (s)", y="Time All ON (s)") -> (x+y=w959:u32)
                    n190 = To Double Precision Float(number=w959) -> (double precision float=w958:dbl)
                    n191 = Divide(x=w958, y=60.0) -> (x/y=w960:dbl)
                    n192 = case shown="False" w977 {
                      tunnel: [w1016 w1032] -> w978
                      tunnel: [w1017 w1024] -> w964
                      tunnel: w975 -> [w1017 w1031]
                      tunnel: w976 -> [w1016 w1030]
                      tunnel: w973 -> [_ w1029]
                      tunnel: [w1015 w1027] -> w966
                      tunnel: w960 -> [_ w1021]
                      tunnel: "Time All OFF (s)" -> [_ w1019]
                      tunnel: "Time All ON (s)" -> [_ w1018]
                      frame False {
                        n193 = Number To Engineering String(4:"HD/CYC Temp") -> (0:w1015:string)  [unwired: 3 in]
                      }
                      frame True {
                        n194 = Divide(x=w1029, y=w1021) -> (x/y=w1028:dbl)
                        n195 = call "WSVCAP SHL Host TL RFFE Write - Multiple DUTs - Common Data.vi"("Data Out"="070201000000", "error in"=w1031, "Log (T)"=FALSE) -> ("error out"=w1034:errorcluster)  [unwired: 12 in]
                        n196 = Round To Nearest(number=w1028) -> (nearest integer value=w1023:dbl)
                        n197 = call "Delay.vi"("milliseconds to wait"=u32 50, "error in (no error)"=w1034) -> ("error out"=w1025:errorcluster)  [unwired: 9 in]
                        n198 = To Long Integer(number=w1023) -> (32bit integer=w1022:i32)
                        "No LPs to RP" <- w1022
                        n199 = for {
                          N: w1022 -> [_]
                          tunnel: w1030 -> [w1052]
                          tunnel: [w1051] -> w1032
                          tunnel: w1025 -> [w1041]
                          tunnel: [w1040] -> w1024
                          tunnel: w1019 -> [w1038]
                          tunnel: w1018 -> [w1036]
                          i -> [w1050]
                          stop <- w1051 stop-if-true
                          w1039 = FALSE ("Log (T)")
                          w1037 = u32 1 ("milliseconds to wait")
                          n200 = Increment(x=w1050) -> (x+1=→"LPs Count":i32)
                          n201 = call "WSVCAP SHL Host TL RFFE Write - Multiple DUTs - Common Data.vi"("Data Out"="074776", "error in"=w1041, "Log (T)"=w1039) -> ("error out"=w1058:errorcluster)  [unwired: 12 in]
                          n202 = call "Delay.vi"("milliseconds to wait"=w1037, "error in (no error)"=w1058) -> ("error out"=w1057:errorcluster)  [unwired: 9 in]
                          n203 = local read "CP to HD/Cycle"() -> (w1043:i32)
                          n204 = call "WSVCAP SHL Host TL RFFE Write - Multiple DUTs - Common Data.vi"("Data Out"="070201000000", "error in"=w1044) -> ("error out"=w1054:errorcluster)  [unwired: 13 in]
                          n205 = call "WSVCAP SHL Host TL RFFE Write - Multiple DUTs - Common Data.vi"("Data Out"="0702013B3B3B", "error in"=w1057, "Log (T)"=w1039) -> ("error out"=w1047:errorcluster)  [unwired: 12 in]
                          n206 = call "Delay.vi"("milliseconds to wait"=w1037, "error in (no error)"=w1047) -> ("error out"=w1046:errorcluster)  [unwired: 9 in]
                          n207 = flat-sequence {
                            tunnel: w1054 -> [w1065]
                            tunnel: [w1063] -> w1040
                            tunnel: w1038 -> [w1060]
                            frame #0 {
                              n208 = local write "STATUS"("Now HD OFF Time..." ("STATUS")) -> ()
                              n209 = Multiply(x=w1060, y=u32 1000) -> (x*y=w1062:u32)
                              n210 = call "Delay.vi"("milliseconds to wait"=w1062, "error in (no error)"=w1065) -> ("error out"=w1063:errorcluster)  [unwired: 9 in]
                            }
                          }
                          n211 = Index Array(array=string[] ["07476F", "074776", "074765", "074769", "07477B"], index=w1043) -> (element=w1048:string)
                          n212 = call "WSVCAP SHL Host TL RFFE Write - Multiple DUTs - Common Data.vi"("Data Out"=w1048, "error in"=w1046, "Log (T)"=w1039) -> ("error out"=w1045:errorcluster)  [unwired: 12 in]
                          n213 = flat-sequence {
                            tunnel: [w1070] -> w1044
                            tunnel: w1045 -> [w1067]
                            tunnel: w1036 -> [w1066]
                            frame #0 {
                              n214 = local write "STATUS"("Now HD ON Time..." ("STATUS")) -> ()
                              n215 = Multiply(x=w1066, y=u32 1000) -> (x*y=w1069:u32)
                              n216 = call "Delay.vi"("milliseconds to wait"=w1069, "error in (no error)"=w1067) -> ("error out"=w1070:errorcluster)  [unwired: 9 in]
                            }
                          }
                          n217 = Unbundle By Name(w1040) -> ("status"=w1053:bool)
                          n218 = Or(x=w1053, y=w1052) -> (x .or. y?=w1051:bool)
                        }
                        n219 = Number To Engineering String(4:"DC_Temp") -> (0:w1027:string)  [unwired: 3 in]
                      }
                    }
                  }
                }
                n220 = case shown="0, Default" "CP to Meas" {
                  selector: "CP to Meas" -> [w776 w781 w786 w791 w796 w801 w806 w811 w815]
                  tunnel: string[] ["07476F", "074776", "074765", "074769", "07477B", "07477C", "07477D", "074779", "07476B"] -> [w777 w782 w787 w792 w797 w802 w807 w812 w817]
                  tunnel: [w775 w780 w785 w790 w795 w800 w805 w810 w816] -> w686
                  tunnel: ["35.0" ("Data Out") "27.5" ("Data Out") "30.5" ("Data Out") "44.0" ("Data Out") "50.0" ("Data Out") "55.0" ("Data Out") "42.5" ("Data Out") "32.0" ("Data Out") "40.25" ("Data Out")] -> w690
                  tunnel: [w773 w778 w783 w788 w793 w798 w803 w808 w813] -> w689
                  tunnel: w688 -> [w773 w778 w783 w788 w793 w798 w803 w808 w813]
                  frame 0, Default {
                    n221 = Index Array(array=w777, index=w776) -> (element=w775:string)
                  }
                  frame 2 {
                    n222 = Index Array(array=w782, index=w781) -> (element=w780:string)
                  }
                  frame 3 {
                    n223 = Index Array(array=w787, index=w786) -> (element=w785:string)
                  }
                  frame 4 {
                    n224 = Index Array(array=w792, index=w791) -> (element=w790:string)
                  }
                  frame 5 {
                    n225 = Index Array(array=w797, index=w796) -> (element=w795:string)
                  }
                  frame 6 {
                    n226 = Index Array(array=w802, index=w801) -> (element=w800:string)
                  }
                  frame 7 {
                    n227 = Index Array(array=w807, index=w806) -> (element=w805:string)
                  }
                  frame 8 {
                    n228 = Index Array(array=w812, index=w811) -> (element=w810:string)
                  }
                  frame 1 {
                    n229 = Index Array(array=w817, index=w815) -> (element=w816:string)
                  }
                }
                n230 = call "WSVCAP SHL Host TL RFFE Write - Multiple DUTs - Common Data.vi"("Data Out"=w686, "error in"=w689, "Log (T)"=w712) -> ("error out"=w728:errorcluster)  [unwired: 12 in]
                n231 = flat-sequence {
                  tunnel: w714 -> [w831]
                  tunnel: [w831] -> w710
                  frame #0 {
                    w833 = "0" ("NOM IDD OFF(uA)")
                    w834 = string[] []
                    w835 = string[][] []
                    n232 = To Long Integer(number=0.0 ("No of Loops to RP")) -> (32bit integer=w832:i32)
                    n233 = local write "NOM IDD ON (uA)"(w833) -> ()
                    n234 = local write "NOM IDD OFF(uA)"(w833) -> ()
                    n235 = local write "LPs Count"(w832) -> ()
                    n236 = local write "No LPs to RP"(w832) -> ()
                    n237 = local write "Total Delta C1(pF)"(w834) -> ()
                    n238 = local write "Total Delta C2(pF)"(w834) -> ()
                    n239 = local write "Total Delta C3(pF)"(w834) -> ()
                    n240 = local write "Current EFuse Read back"(w834) -> ()
                    n241 = local write "RB Reg for HD"(w834) -> ()
                    n242 = local write "RB Reg for HD/Cycle"(w834) -> ()
                    n243 = local write "CAP_C3"(w835) -> ()
                    n244 = local write "CAP_C2"(w835) -> ()
                    n245 = local write "CAP_C1"(w835) -> ()
                    n246 = local write "VSA_V3"(w835) -> ()
                    n247 = local write "VSA_V1"(w835) -> ()
                    n248 = local write "VSA_V2"(w835) -> ()
                    n249 = local write "VPI C1"(w835) -> ()
                    n250 = local write "VPI C2"(w835) -> ()
                    n251 = local write "VPI C3"(w835) -> ()
                    n252 = local write "% Delta C"(w835) -> ()
                  }
                }
                n253 = call "Delay.vi"("milliseconds to wait"=u32 50, "error in (no error)"=w728) -> ("error out"=w694:errorcluster)  [unwired: 9 in]
                n254 = for {
                  tunnel: [w830] -> w739
                  tunnel: [w829] -> w714
                  tunnel: w712 -> [w828]
                  tunnel: w701 -> [w827]
                  tunnel: w694 -> [w823]
                  tunnel: string[] ["0702013B3B3B", "070201000000"] -> [w819] mode=indexing
                  tunnel: [w818] -> w697 mode=indexing
                  n255 = call "WSVCAP SHL Host TL RFFE Write - Multiple DUTs - Common Data.vi"("Data Out"=w819, "error in"=w823, "Log (T)"=w828) -> ("error out"=w824:errorcluster)  [unwired: 12 in]
                  n256 = local read "IDD Brd(uA)"() -> (w820:string)
                  n257 = call "Delay.vi"("milliseconds to wait"=u32 100, "error in (no error)"=w824) -> ("error out"=w825:errorcluster)  [unwired: 9 in]
                  n258 = call "Ke2000 Single Reading.vi"("error in (no error)"=w825, "VISA resource name"=w827) -> ("error out"=w822:errorcluster, "VISA resource name out"=w830:refnum<visa-resource-name>, "uA"=w821:string)  [unwired: 5 in, 2 out]
                  n259 = call "Substration.vi"("error in (no error)"=w822, "Input2"=w820, "Input1"=w821) -> ("error out"=w829:errorcluster, "In1 - In2"=w818:string)  [unwired: 7 in]
                }
                n260 = Index Array(array=w697, index=1) -> (element=w696:string)
                n261 = Index Array(array=w697, index=0) -> (element=w699:string)
                n262 = local read "Clock Rate (Hz)"() -> (w729:dbl)
                n263 = call "Multi Dut Cmd_Header Setting.vi"("WS1050/51"="WS1050/51", "Cmin/Act"="Cmin/Act", "Test Seq"="Test Sequences", "error in (no error)"=w710) -> ("Name 1"=w708:string[], "Name 2"=w707:string[], "Name Header"=w705:string[], "Name 3"=w706:string[], "Cmd 3"=w702:string[], "Cmd 1"=w704:string[], "Cmd 2"=w703:string[], "error out"=w711:errorcluster)  [unwired: 2 in, 2 out]
              }
              frame #1 {
                w1081 = FALSE ("Log (T)")
                n264 = call "WSVCAP SHL Host TL RFFE Configure.vi"("RFFE Slave Address"=w1092, "Clock Rate (Hz)"=w1090, "error in"=w1082) -> ("Actual Rate (Hz)"=w1100:dbl, "error out"=w1088:errorcluster)  [unwired: 11 in]
                n265 = local write "AR  Measurent(Hz)"(w1100) -> ()
                n266 = Array Size(array=w1093) -> (size(s)=w1103:i32)
                n267 = case shown="False" w1072 {
                  tunnel: w1103 -> [w1111 _]
                  tunnel: w1094 -> [w1110 _]
                  tunnel: w1093 -> [w1109 _]
                  tunnel: w1088 -> [w1108 w1197]
                  tunnel: [w1107 w1197] -> w1087
                  tunnel: w1081 -> [w1106 _]
                  tunnel: [w1105 string[][] []] -> w1076
                  tunnel: w1075 -> [w1104 _]
                  frame False {
                    n268 = case shown="2" w1104 {
                      tunnel: w1111 -> [w1118 w1146 w1174]
                      tunnel: w1110 -> [w1117 w1145 w1173]
                      tunnel: w1109 -> [w1116 w1144 w1172]
                      tunnel: w1108 -> [w1115 w1143 w1171]
                      tunnel: [w1114 w1142 w1170] -> w1107
                      tunnel: w1106 -> [w1113 w1141 w1169]
                      tunnel: [w1112 w1140 w1168] -> w1105
                      frame 0, Default {
                        n269 = for {
                          N: w1118 -> [_]
                          tunnel: w1117 -> [w1135]
                          tunnel: [w1131] -> w1112 mode=indexing
                          tunnel: w1116 -> [w1133]
                          tunnel: w1115 -> [w1121]
                          tunnel: [w1123] -> w1114
                          tunnel: w1113 -> [w1122]
                          i -> [w1130]
                          stop <- w1119 stop-if-true
                          n270 = Index Array(array=w1135, index=w1130) -> (element=w1134:string)
                          n271 = Index Array(array=w1133, index=w1130) -> (element=w1132:string)
                          n272 = local write "STATUS"(w1132) -> ()
                          n273 = call "WSVCAP SHL Host TL RFFE Write - Multiple DUTs - Common Data.vi"("Data Out"=w1134, "error in"=w1121, "Log (T)"=FALSE) -> ("error out"=w1125:errorcluster)  [unwired: 12 in]
                          n274 = call "Delay.vi"("milliseconds to wait"=u32 10, "error in (no error)"=w1125) -> ("error out"=w1129:errorcluster)  [unwired: 9 in]
                          n275 = call "WS1050 AD7747 READ 36 DUT.vi"("error in"=w1129, "Log (T)"=w1122, "DUT Mask Mode (All)"=WSVCAP_SHL_I2C_DUT_Mask_Mode_Enum."C1") -> ("error out"=w1127:errorcluster, "AD7747 Values"=w1128:string[][])  [unwired: 7 in]
                          n276 = for {
                            tunnel: w1128 -> [w1138] mode=indexing
                            tunnel: w1127 -> [w1139]
                            tunnel: [w1139] -> w1123
                            tunnel: [w1136] -> w1131 mode=indexing
                            n277 = Index Array(array=w1138, index=1) -> (element=w1136:string)
                          }
                          n278 = Unbundle By Name(w1123) -> ("status"=w1119:bool)
                        }
                      }
                      frame 1 {
                        n279 = for {
                          N: w1146 -> [_]
                          tunnel: w1145 -> [w1163]
                          tunnel: [w1159] -> w1140 mode=indexing
                          tunnel: w1144 -> [w1161]
                          tunnel: w1143 -> [w1149]
                          tunnel: [w1151] -> w1142
                          tunnel: w1141 -> [w1150]
                          i -> [w1158]
                          stop <- w1147 stop-if-true
                          n280 = Index Array(array=w1163, index=w1158) -> (element=w1162:string)
                          n281 = Index Array(array=w1161, index=w1158) -> (element=w1160:string)
                          n282 = local write "STATUS"(w1160) -> ()
                          n283 = call "WSVCAP SHL Host TL RFFE Write - Multiple DUTs - Common Data.vi"("Data Out"=w1162, "error in"=w1149, "Log (T)"=FALSE) -> ("error out"=w1153:errorcluster)  [unwired: 12 in]
                          n284 = call "Delay.vi"("milliseconds to wait"=u32 10, "error in (no error)"=w1153) -> ("error out"=w1157:errorcluster)  [unwired: 9 in]
                          n285 = call "WS1050 AD7747 READ 36 DUT.vi"("error in"=w1157, "Log (T)"=w1150, "DUT Mask Mode (All)"=WSVCAP_SHL_I2C_DUT_Mask_Mode_Enum."C2") -> ("error out"=w1155:errorcluster, "AD7747 Values"=w1156:string[][])  [unwired: 7 in]
                          n286 = for {
                            tunnel: w1156 -> [w1166] mode=indexing
                            tunnel: w1155 -> [w1167]
                            tunnel: [w1167] -> w1151
                            tunnel: [w1164] -> w1159 mode=indexing
                            n287 = Index Array(array=w1166, index=3) -> (element=w1164:string)
                          }
                          n288 = Unbundle By Name(w1151) -> ("status"=w1147:bool)
                        }
                      }
                      frame 2 {
                        n289 = for {
                          N: w1174 -> [_]
                          tunnel: w1173 -> [w1191]
                          tunnel: [w1187] -> w1168 mode=indexing
                          tunnel: w1172 -> [w1189]
                          tunnel: w1171 -> [w1177]
                          tunnel: [w1179] -> w1170
                          tunnel: w1169 -> [w1178]
                          i -> [w1186]
                          stop <- w1175 stop-if-true
                          n290 = Index Array(array=w1191, index=w1186) -> (element=w1190:string)
                          n291 = Index Array(array=w1189, index=w1186) -> (element=w1188:string)
                          n292 = local write "STATUS"(w1188) -> ()
                          n293 = call "WSVCAP SHL Host TL RFFE Write - Multiple DUTs - Common Data.vi"("Data Out"=w1190, "error in"=w1177, "Log (T)"=FALSE) -> ("error out"=w1181:errorcluster)  [unwired: 12 in]
                          n294 = call "Delay.vi"("milliseconds to wait"=u32 10, "error in (no error)"=w1181) -> ("error out"=w1185:errorcluster)  [unwired: 9 in]
                          n295 = call "WS1050 AD7747 READ 36 DUT.vi"("error in"=w1185, "Log (T)"=w1178, "DUT Mask Mode (All)"=WSVCAP_SHL_I2C_DUT_Mask_Mode_Enum."C3") -> ("error out"=w1183:errorcluster, "AD7747 Values"=w1184:string[][])  [unwired: 7 in]
                          n296 = for {
                            tunnel: w1184 -> [w1194] mode=indexing
                            tunnel: w1183 -> [w1195]
                            tunnel: [w1195] -> w1179
                            tunnel: [w1192] -> w1187 mode=indexing
                            n297 = Index Array(array=w1194, index=5) -> (element=w1192:string)
                          }
                          n298 = Unbundle By Name(w1179) -> ("status"=w1175:bool)
                        }
                      }
                    }
                  }
                  frame True {
                  }
                }
                n299 = Transpose 2D Array(2D array=w1076) -> (transposed array=w1086:string[][])
                "CAP_C1" <- w1086
                "NOM IDD ON (uA)" <- w1096
                "NOM IDD OFF(uA)" <- w1095
              }
              frame #2 {
                n300 = Array Size(array=w1215) -> (size(s)=w1216:i32)
                n301 = case shown="True" w1198 {
                  tunnel: w1216 -> [w1232 _]
                  tunnel: w1215 -> [w1231 _]
                  tunnel: w1214 -> [w1230 _]
                  tunnel: [w1229 w1290] -> w1212
                  tunnel: w1210 -> [w1228 w1290]
                  tunnel: w1204 -> [w1227 _]
                  tunnel: [w1226 string[][] []] -> w1202
                  tunnel: w1201 -> [w1225 _]
                  frame False {
                    n302 = case shown="0, 2, Default" w1225 {
                      tunnel: w1232 -> [w1239 w1267]
                      tunnel: w1231 -> [w1238 w1266]
                      tunnel: w1230 -> [w1237 w1265]
                      tunnel: [w1236 w1264] -> w1229
                      tunnel: w1228 -> [w1235 w1263]
                      tunnel: w1227 -> [w1234 w1262]
                      tunnel: [w1233 w1261] -> w1226
                      frame 0, 2, Default {
                        n303 = for {
                          N: w1239 -> [_]
                          tunnel: w1237 -> [w1256]
                          tunnel: [w1252] -> w1233 mode=indexing
                          tunnel: w1238 -> [w1254]
                          tunnel: w1235 -> [w1242]
                          tunnel: [w1244] -> w1236
                          tunnel: w1234 -> [w1243]
                          i -> [w1251]
                          stop <- w1240 stop-if-true
                          n304 = Index Array(array=w1256, index=w1251) -> (element=w1255:string)
                          n305 = Index Array(array=w1254, index=w1251) -> (element=w1253:string)
                          n306 = call "WSVCAP SHL Host TL RFFE Write - Multiple DUTs - Common Data.vi"("Data Out"=w1255, "error in"=w1242, "Log (T)"=FALSE) -> ("error out"=w1246:errorcluster)  [unwired: 12 in]
                          n307 = local write "STATUS"(w1253) -> ()
                          n308 = call "Delay.vi"("milliseconds to wait"=u32 10, "error in (no error)"=w1246) -> ("error out"=w1250:errorcluster)  [unwired: 9 in]
                          n309 = call "WS1050 AD7747 READ 36 DUT.vi"("error in"=w1250, "Log (T)"=w1243, "DUT Mask Mode (All)"=WSVCAP_SHL_I2C_DUT_Mask_Mode_Enum."C2") -> ("error out"=w1248:errorcluster, "AD7747 Values"=w1249:string[][])  [unwired: 7 in]
                          n310 = for {
                            tunnel: w1249 -> [w1259] mode=indexing
                            tunnel: w1248 -> [w1260]
                            tunnel: [w1260] -> w1244
                            tunnel: [w1257] -> w1252 mode=indexing
                            n311 = Index Array(array=w1259, index=3) -> (element=w1257:string)
                          }
                          n312 = Unbundle By Name(w1244) -> ("status"=w1240:bool)
                        }
                      }
                      frame 1 {
                        n313 = for {
                          N: w1267 -> [_]
                          tunnel: w1265 -> [w1284]
                          tunnel: [w1280] -> w1261 mode=indexing
                          tunnel: w1266 -> [w1282]
                          tunnel: w1263 -> [w1270]
                          tunnel: [w1272] -> w1264
                          tunnel: w1262 -> [w1271]
                          i -> [w1279]
                          stop <- w1268 stop-if-true
                          n314 = Index Array(array=w1284, index=w1279) -> (element=w1283:string)
                          n315 = Index Array(array=w1282, index=w1279) -> (element=w1281:string)
                          n316 = call "WSVCAP SHL Host TL RFFE Write - Multiple DUTs - Common Data.vi"("Data Out"=w1283, "error in"=w1270, "Log (T)"=FALSE) -> ("error out"=w1274:errorcluster)  [unwired: 12 in]
                          n317 = local write "STATUS"(w1281) -> ()
                          n318 = call "Delay.vi"("milliseconds to wait"=u32 10, "error in (no error)"=w1274) -> ("error out"=w1278:errorcluster)  [unwired: 9 in]
                          n319 = call "WS1050 AD7747 READ 36 DUT.vi"("error in"=w1278, "Log (T)"=w1271, "DUT Mask Mode (All)"=WSVCAP_SHL_I2C_DUT_Mask_Mode_Enum."C1") -> ("error out"=w1276:errorcluster, "AD7747 Values"=w1277:string[][])  [unwired: 7 in]
                          n320 = for {
                            tunnel: w1277 -> [w1287] mode=indexing
                            tunnel: w1276 -> [w1288]
                            tunnel: [w1288] -> w1272
                            tunnel: [w1285] -> w1280 mode=indexing
                            n321 = Index Array(array=w1287, index=1) -> (element=w1285:string)
                          }
                          n322 = Unbundle By Name(w1272) -> ("status"=w1268:bool)
                        }
                      }
                    }
                  }
                  frame True {
                  }
                }
                n323 = Transpose 2D Array(2D array=w1202) -> (transposed array=w1211:string[][])
                "CAP_C2" <- w1211
              }
              frame #3 {
                n324 = Array Size(array=w1308) -> (size(s)=w1309:i32)
                n325 = case shown="True" w1291 {
                  tunnel: w1309 -> [w1326 _]
                  tunnel: w1308 -> [w1325 _]
                  tunnel: w1307 -> [w1324 _]
                  tunnel: w1302 -> [w1323 w1384]
                  tunnel: w1298 -> [w1322 _]
                  tunnel: [w1321 string[][] []] -> w1296
                  tunnel: w1295 -> [w1320 _]
                  tunnel: [w1319 w1384] -> w1294
                  frame False {
                    n326 = case shown="2" w1320 {
                      tunnel: w1326 -> [w1333 w1361]
                      tunnel: w1325 -> [w1332 w1360]
                      tunnel: w1324 -> [w1331 w1359]
                      tunnel: w1323 -> [w1330 w1358]
                      tunnel: [w1329 w1357] -> w1319
                      tunnel: w1322 -> [w1328 w1356]
                      tunnel: [w1327 w1355] -> w1321
                      frame 0, 1, Default {
                        n327 = for {
                          N: w1333 -> [_]
                          tunnel: w1331 -> [w1350]
                          tunnel: [w1346] -> w1327 mode=indexing
                          tunnel: w1332 -> [w1348]
                          tunnel: w1330 -> [w1336]
                          tunnel: [w1338] -> w1329
                          tunnel: w1328 -> [w1337]
                          i -> [w1345]
                          stop <- w1334 stop-if-true
                          n328 = Index Array(array=w1350, index=w1345) -> (element=w1349:string)
                          n329 = Index Array(array=w1348, index=w1345) -> (element=w1347:string)
                          n330 = local write "STATUS"(w1347) -> ()
                          n331 = call "WSVCAP SHL Host TL RFFE Write - Multiple DUTs - Common Data.vi"("Data Out"=w1349, "error in"=w1336, "Log (T)"=FALSE) -> ("error out"=w1340:errorcluster)  [unwired: 12 in]
                          n332 = call "Delay.vi"("milliseconds to wait"=u32 10, "error in (no error)"=w1340) -> ("error out"=w1344:errorcluster)  [unwired: 9 in]
                          n333 = call "WS1050 AD7747 READ 36 DUT.vi"("error in"=w1344, "Log (T)"=w1337, "DUT Mask Mode (All)"=WSVCAP_SHL_I2C_DUT_Mask_Mode_Enum."C3") -> ("error out"=w1342:errorcluster, "AD7747 Values"=w1343:string[][])  [unwired: 7 in]
                          n334 = for {
                            tunnel: w1343 -> [w1353] mode=indexing
                            tunnel: w1342 -> [w1354]
                            tunnel: [w1354] -> w1338
                            tunnel: [w1351] -> w1346 mode=indexing
                            n335 = Index Array(array=w1353, index=5) -> (element=w1351:string)
                          }
                          n336 = Unbundle By Name(w1338) -> ("status"=w1334:bool)
                        }
                      }
                      frame 2 {
                        n337 = for {
                          N: w1361 -> [_]
                          tunnel: w1359 -> [w1378]
                          tunnel: [w1374] -> w1355 mode=indexing
                          tunnel: w1360 -> [w1376]
                          tunnel: w1358 -> [w1364]
                          tunnel: [w1366] -> w1357
                          tunnel: w1356 -> [w1365]
                          i -> [w1373]
                          stop <- w1362 stop-if-true
                          n338 = Index Array(array=w1378, index=w1373) -> (element=w1377:string)
                          n339 = Index Array(array=w1376, index=w1373) -> (element=w1375:string)
                          n340 = local write "STATUS"(w1375) -> ()
                          n341 = call "WSVCAP SHL Host TL RFFE Write - Multiple DUTs - Common Data.vi"("Data Out"=w1377, "error in"=w1364, "Log (T)"=FALSE) -> ("error out"=w1368:errorcluster)  [unwired: 12 in]
                          n342 = call "Delay.vi"("milliseconds to wait"=u32 10, "error in (no error)"=w1368) -> ("error out"=w1372:errorcluster)  [unwired: 9 in]
                          n343 = call "WS1050 AD7747 READ 36 DUT.vi"("error in"=w1372, "Log (T)"=w1365, "DUT Mask Mode (All)"=WSVCAP_SHL_I2C_DUT_Mask_Mode_Enum."C1") -> ("error out"=w1370:errorcluster, "AD7747 Values"=w1371:string[][])  [unwired: 7 in]
                          n344 = for {
                            tunnel: w1371 -> [w1381] mode=indexing
                            tunnel: w1370 -> [w1382]
                            tunnel: [w1382] -> w1366
                            tunnel: [w1379] -> w1374 mode=indexing
                            n345 = Index Array(array=w1381, index=1) -> (element=w1379:string)
                          }
                          n346 = Unbundle By Name(w1366) -> ("status"=w1362:bool)
                        }
                      }
                    }
                  }
                  frame True {
                  }
                }
                n347 = Transpose 2D Array(2D array=w1296) -> (transposed array=w1303:string[][])
                "CAP_C3" <- w1303
              }
              frame #4 {
                # "VPI Testing @ 35V"
                n348 = call "WS1050 Delta C Calculation.vi"("error in (no error)"=w1426, "DCap Target(pF)"=w1425, "Input"=w1428) -> ("error out"=w1423:errorcluster, "Total Bank Delta C(pF)"=w1416:string[], "% Bank DeltaC"=w1420:string[])  [unwired: 3 in, 3 out]
                n349 = call "WS1050 Delta C Calculation.vi"("error in (no error)"=w1426, "DCap Target(pF)"=w1425, "Input"=w1427) -> ("error out"=w1424:errorcluster, "Total Bank Delta C(pF)"=w1415:string[], "% Bank DeltaC"=w1418:string[])  [unwired: 3 in, 3 out]
                n350 = call "WS1050 Delta C Calculation.vi"("error in (no error)"=w1426, "DCap Target(pF)"=w1425, "Input"=w1419) -> ("error out"=w1422:errorcluster, "Total Bank Delta C(pF)"=w1414:string[], "% Bank DeltaC"=w1417:string[])  [unwired: 3 in, 3 out]
                n351 = Merge Errors(w1423, w1424, w1422) -> (w1421:errorcluster)
                n352 = case shown="1, Default" w1429 {
                  tunnel: w1421 -> [w1627 w1635]
                  tunnel: [w1627 w1635] -> w1388
                  tunnel: w1420 -> [w1623 w1631]
                  tunnel: w1418 -> [w1622 w1630]
                  tunnel: w1417 -> [w1621 w1629]
                  tunnel: w1416 -> [w1626 w1634]
                  tunnel: [w1626 w1634] -> w1413
                  tunnel: w1415 -> [w1625 w1633]
                  tunnel: [w1625 w1633] -> w1412
                  tunnel: w1414 -> [w1624 w1632]
                  tunnel: [w1624 w1632] -> w1411
                  frame 0 {
                    n353 = Build Array(w1623, w1622, w1621) -> (→"% Delta C_T0":string[][])
                  }
                  frame 1, Default {
                    n354 = Build Array(w1631, w1630, w1629) -> (→"% Delta C":string[][])
                  }
                }
                "Total Delta C1(pF)" <- w1413
                "Total Delta C2(pF)" <- w1412
                "Total Delta C3(pF)" <- w1411
                n355 = call "WS1050_51 VPI Header.vi"("VPI Name"="VPI Name", "VPI_Cmd"="VPI_Cmd", "Cmin/Act"=w1386, "WS1050/51"=w1397, "error in (no error)"=w1398) -> ("VPI_1"=w1396:string[], "VPI_2"=w1394:string[], "VPI Header"=w1395:string[], "VPI_3"=w1393:string[], "Cmd_3"=w1390:string[], "Cmd_1"=w1392:string[], "Cmd_2"=w1391:string[], "error out"=w1389:errorcluster)  [unwired: 3 in]
                n356 = Merge Errors(w1389, w1388) -> (w1387:errorcluster)
                n357 = case shown="False" w1385 {
                  tunnel: [w1456 w1611] -> w1441
                  tunnel: [w1455 w1611] -> w1440
                  tunnel: w1436 -> [w1454 w1609]
                  tunnel: [w1453 w1609] -> w1435
                  tunnel: [w1452 w1611] -> w1432
                  tunnel: [w1451 "" ("Data Out")] -> w1409
                  tunnel: [w1450 w1610] -> w1407
                  tunnel: w1403 -> [w1449 _]
                  tunnel: w1396 -> [w1448 _]
                  tunnel: w1394 -> [w1447 _]
                  tunnel: w1393 -> [w1446 _]
                  tunnel: w1392 -> [w1445 _]
                  tunnel: w1391 -> [w1444 _]
                  tunnel: w1390 -> [w1443 _]
                  tunnel: w1387 -> [w1442 w1610]
                  frame False {
                    n358 = case shown="False" w1449 {
                      tunnel: [w1459 w1480] -> w1450
                      tunnel: [w1457 w1498] -> w1456
                      tunnel: [w1457 w1484] -> w1455
                      tunnel: w1454 -> [w1464 w1497]
                      tunnel: [w1464 w1497] -> w1453
                      tunnel: w1445 -> [_ w1496]
                      tunnel: w1444 -> [_ w1490]
                      tunnel: w1443 -> [_ w1486]
                      tunnel: [w1457 w1495] -> w1452
                      tunnel: w1448 -> [w1462 w1493]
                      tunnel: w1447 -> [_ w1491]
                      tunnel: w1446 -> [_ w1487]
                      tunnel: ["NA" ("string") w1474] -> w1451
                      tunnel: w1442 -> [w1460 w1478]
                      frame False {
                        n359 = Array Size(array=w1462) -> (size(s)=w1461:i32)
                        n360 = for {
                          N: w1461 -> [_]
                          tunnel: [w1466] -> w1458 mode=indexing
                          tunnel: w1460 -> [w1465]
                          tunnel: [w1465] -> w1459
                          n361 = for {
                            N: 36 -> [_]
                            tunnel: [""] -> w1466 mode=indexing
                          }
                        }
                        n362 = Transpose 2D Array(2D array=w1458) -> (transposed array=w1457:string[][])
                        n363 = local write "VPI C1"(w1457) -> ()
                        n364 = local write "VPI C2"(w1457) -> ()
                        n365 = local write "VPI C3"(w1457) -> ()
                      }
                      frame True {
                        w1479 = FALSE ("Log (T)")
                        # "Set CP VPI"
                        n366 = call "WSVCAP SHL Host TL RFFE Write - Multiple DUTs - Common Data.vi"("Data Out"="074820", "error in"=w1478, "Log (T)"=w1479) -> ("error out"=w1476:errorcluster)  [unwired: 12 in]
                        n367 = call "Delay.vi"("milliseconds to wait"=u32 10, "error in (no error)"=w1476) -> ("error out"=w1472:errorcluster)  [unwired: 9 in]
                        n368 = case shown="0, Default" "CP VPI" {
                          selector: "CP VPI" -> [w1503 w1508 w1513 w1518 w1523 w1528 w1533 w1538 w1542]
                          tunnel: string[] ["07476F", "074776", "074765", "074769", "07477B", "07477C", "07477D", "074779", "07476B"] -> [w1504 w1509 w1514 w1519 w1524 w1529 w1534 w1539 w1544]
                          tunnel: [w1502 w1507 w1512 w1517 w1522 w1527 w1532 w1537 w1543] -> w1471
                          tunnel: ["35.0" ("Data Out") "27.5" ("Data Out") "30.5" ("Data Out") "44.0" ("Data Out") "50.0" ("Data Out") "55.0" ("Data Out") "42.5" ("Data Out") "32.0" ("Data Out") "40.25" ("Data Out")] -> w1474
                          tunnel: [w1500 w1505 w1510 w1515 w1520 w1525 w1530 w1535 w1540] -> w1473
                          tunnel: w1472 -> [w1500 w1505 w1510 w1515 w1520 w1525 w1530 w1535 w1540]
                          frame 0, Default {
                            n369 = Index Array(array=w1504, index=w1503) -> (element=w1502:string)
                          }
                          frame 2 {
                            n370 = Index Array(array=w1509, index=w1508) -> (element=w1507:string)
                          }
                          frame 3 {
                            n371 = Index Array(array=w1514, index=w1513) -> (element=w1512:string)
                          }
                          frame 4 {
                            n372 = Index Array(array=w1519, index=w1518) -> (element=w1517:string)
                          }
                          frame 5 {
                            n373 = Index Array(array=w1524, index=w1523) -> (element=w1522:string)
                          }
                          frame 6 {
                            n374 = Index Array(array=w1529, index=w1528) -> (element=w1527:string)
                          }
                          frame 7 {
                            n375 = Index Array(array=w1534, index=w1533) -> (element=w1532:string)
                          }
                          frame 8 {
                            n376 = Index Array(array=w1539, index=w1538) -> (element=w1537:string)
                          }
                          frame 1 {
                            n377 = Index Array(array=w1544, index=w1542) -> (element=w1543:string)
                          }
                        }
                        n378 = Array Size(array=w1493) -> (size(s)=w1499:i32)
                        n379 = call "WSVCAP SHL Host TL RFFE Write - Multiple DUTs - Common Data.vi"("Data Out"=w1471, "error in"=w1473, "Log (T)"=w1479) -> ("error out"=w1483:errorcluster)  [unwired: 12 in]
                        n380 = for {
                          N: w1499 -> [_]
                          tunnel: w1496 -> [w1603]
                          tunnel: [w1601] -> w1494 mode=indexing
                          tunnel: w1493 -> [w1600]
                          tunnel: w1483 -> [w1589]
                          tunnel: [w1591] -> w1482
                          i -> [w1599]
                          stop <- w1587 stop-if-true
                          n381 = Index Array(array=w1603, index=w1599) -> (element=w1602:string)
                          n382 = Index Array(array=w1600, index=w1599) -> (element=w1598:string)
                          n383 = local write "STATUS"(w1598) -> ()
                          n384 = call "WSVCAP SHL Host TL RFFE Write - Multiple DUTs - Common Data.vi"("Data Out"=w1602, "error in"=w1589, "Log (T)"=FALSE) -> ("error out"=w1597:errorcluster)  [unwired: 12 in]
                          n385 = call "Delay.vi"("milliseconds to wait"=u32 10, "error in (no error)"=w1597) -> ("error out"=w1593:errorcluster)  [unwired: 9 in]
                          n386 = call "WS1050 AD7747 READ 36 DUT.vi"("error in"=w1593, "Log (T)"=FALSE, "DUT Mask Mode (All)"=WSVCAP_SHL_I2C_DUT_Mask_Mode_Enum."C1") -> ("error out"=w1595:errorcluster, "AD7747 Values"=w1594:string[][])  [unwired: 7 in]
                          n387 = for {
                            tunnel: [w1606] -> w1601 mode=indexing
                            tunnel: w1595 -> [w1605]
                            tunnel: [w1605] -> w1591
                            tunnel: w1594 -> [w1604] mode=indexing
                            n388 = Index Array(array=w1604, index=1) -> (element=w1606:string)
                          }
                          n389 = Unbundle By Name(w1591) -> ("status"=w1587:bool)
                        }
                        n390 = Transpose 2D Array(2D array=w1494) -> (transposed array=w1498:string[][])
                        "VPI C1" <- w1498
                        n391 = Array Size(array=w1491) -> (size(s)=w1492:i32)
                        n392 = for {
                          N: w1492 -> [_]
                          tunnel: w1490 -> [w1582]
                          tunnel: [w1580] -> w1489 mode=indexing
                          tunnel: w1491 -> [w1579]
                          tunnel: w1482 -> [w1568]
                          tunnel: [w1570] -> w1481
                          i -> [w1578]
                          stop <- w1566 stop-if-true
                          n393 = Index Array(array=w1582, index=w1578) -> (element=w1581:string)
                          n394 = Index Array(array=w1579, index=w1578) -> (element=w1577:string)
                          n395 = call "WSVCAP SHL Host TL RFFE Write - Multiple DUTs - Common Data.vi"("Data Out"=w1581, "error in"=w1568, "Log (T)"=FALSE) -> ("error out"=w1576:errorcluster)  [unwired: 12 in]
                          n396 = local write "STATUS"(w1577) -> ()
                          n397 = call "Delay.vi"("milliseconds to wait"=u32 10, "error in (no error)"=w1576) -> ("error out"=w1572:errorcluster)  [unwired: 9 in]
                          n398 = call "WS1050 AD7747 READ 36 DUT.vi"("error in"=w1572, "Log (T)"=FALSE, "DUT Mask Mode (All)"=WSVCAP_SHL_I2C_DUT_Mask_Mode_Enum."C2") -> ("error out"=w1574:errorcluster, "AD7747 Values"=w1573:string[][])  [unwired: 7 in]
                          n399 = for {
                            tunnel: [w1585] -> w1580 mode=indexing
                            tunnel: w1574 -> [w1584]
                            tunnel: [w1584] -> w1570
                            tunnel: w1573 -> [w1583] mode=indexing
                            n400 = Index Array(array=w1583, index=3) -> (element=w1585:string)
                          }
                          n401 = Unbundle By Name(w1570) -> ("status"=w1566:bool)
                        }
                        n402 = Transpose 2D Array(2D array=w1489) -> (transposed array=w1495:string[][])
                        "VPI C2" <- w1495
                        n403 = Array Size(array=w1487) -> (size(s)=w1488:i32)
                        n404 = for {
                          N: w1488 -> [_]
                          tunnel: w1486 -> [w1561]
                          tunnel: [w1559] -> w1485 mode=indexing
                          tunnel: w1487 -> [w1558]
                          tunnel: w1481 -> [w1547]
                          tunnel: [w1549] -> w1480
                          i -> [w1557]
                          stop <- w1545 stop-if-true
                          n405 = Index Array(array=w1561, index=w1557) -> (element=w1560:string)
                          n406 = Index Array(array=w1558, index=w1557) -> (element=w1556:string)
                          n407 = call "WSVCAP SHL Host TL RFFE Write - Multiple DUTs - Common Data.vi"("Data Out"=w1560, "error in"=w1547, "Log (T)"=FALSE) -> ("error out"=w1555:errorcluster)  [unwired: 12 in]
                          n408 = local write "STATUS"(w1556) -> ()
                          n409 = call "Delay.vi"("milliseconds to wait"=u32 10, "error in (no error)"=w1555) -> ("error out"=w1551:errorcluster)  [unwired: 9 in]
                          n410 = call "WS1050 AD7747 READ 36 DUT.vi"("error in"=w1551, "Log (T)"=FALSE, "DUT Mask Mode (All)"=WSVCAP_SHL_I2C_DUT_Mask_Mode_Enum."C3") -> ("error out"=w1553:errorcluster, "AD7747 Values"=w1552:string[][])  [unwired: 7 in]
                          n411 = for {
                            tunnel: [w1564] -> w1559 mode=indexing
                            tunnel: w1553 -> [w1563]
                            tunnel: [w1563] -> w1549
                            tunnel: w1552 -> [w1562] mode=indexing
                            n412 = Index Array(array=w1562, index=5) -> (element=w1564:string)
                          }
                          n413 = Unbundle By Name(w1549) -> ("status"=w1545:bool)
                        }
                        n414 = Transpose 2D Array(2D array=w1485) -> (transposed array=w1484:string[][])
                        "VPI C3" <- w1484
                      }
                    }
                  }
                  frame True {
                    w1611 = string[][] []
                  }
                }
                n415 = Insert Into Array(array=w1431, new element=w1395) -> (w1430:string[])  [unwired: 1 in]
                n416 = case shown="True" w1408 {
                  tunnel: w1407 -> [w1613 w1618]
                  tunnel: [w1614 w1617] -> w1406
                  frame False {
                    n417 = call "WSVCAP SHL Host TL RFFE Write - Multiple DUTs - Common Data.vi"("Data Out"="074820", "error in"=w1613, "Log (T)"=FALSE) -> ("error out"=w1614:errorcluster)  [unwired: 12 in]
                  }
                  frame True {
                    n418 = call "WSVCAP SHL Host TL RFFE Write - Multiple DUTs - Common Data.vi"("Data Out"="074800", "error in"=w1618, "Log (T)"=FALSE) -> ("error out"=w1617:errorcluster)  [unwired: 12 in]
                  }
                }
                n419 = call "Delay.vi"("milliseconds to wait"=u32 10, "error in (no error)"=w1406) -> ("error out"=w1405:errorcluster)  [unwired: 9 in]
              }
              frame #5 {
                # "VSA Testing"
                n420 = case shown="True" w1636 {
                  tunnel: w1676 -> [w1686 w1756]
                  tunnel: w1667 -> [w1685 w1755]
                  tunnel: [w1684 w1755] -> w1666
                  tunnel: [w1683 string[][] []] -> w1656
                  tunnel: [w1682 w1757] -> w1655
                  tunnel: [w1681 w1757] -> w1652
                  tunnel: [w1680 w1756] -> w1650
                  tunnel: [w1679 w1757] -> w1649
                  tunnel: w1637 -> [w1678 _]
                  frame False {
                    n421 = case shown="True" w1678 {
                      tunnel: w1686 -> [w1688 w1702]
                      tunnel: [w1687 w1701] -> w1680
                      tunnel: [w1692 w1708] -> w1684
                      tunnel: w1685 -> [w1692 w1707]
                      tunnel: [w1689 w1705] -> w1682
                      tunnel: [w1689 w1704] -> w1681
                      tunnel: [w1689 w1703] -> w1679
                      tunnel: [w1690 w1706] -> w1683
                      frame False {
                        n422 = for {
                          tunnel: dbl[] [0.0, 0.0, 0.0] -> [w1697] mode=indexing
                          tunnel: [w1696] -> w1690 mode=indexing
                          tunnel: [w1693] -> w1689 mode=indexing
                          tunnel: w1688 -> [w1694]
                          tunnel: [w1694] -> w1687
                          n423 = Number To Fractional String(number=w1697) -> (F-format string=w1698:string)  [unwired: 3 in]
                          n424 = for {
                            N: 36 -> [_]
                            tunnel: w1698 -> [w1700]
                            tunnel: [w1700] -> w1696 mode=indexing
                            tunnel: [""] -> w1693 mode=indexing
                          }
                        }
                      }
                      frame True {
                        n425 = for {
                          tunnel: "VSA Voltage(V)" -> [w1732] mode=indexing
                          tunnel: [w1736] -> w1708
                          tunnel: w1707 -> [w1734]
                          tunnel: [w1733] -> w1705 mode=indexing
                          tunnel: [w1720] -> w1704 mode=indexing
                          tunnel: [w1729] -> w1706 mode=indexing
                          tunnel: [w1714] -> w1703 mode=indexing
                          tunnel: w1702 -> [w1713]
                          tunnel: [w1712] -> w1701
                          w1711 = FALSE ("Log (T)")
                          w1728 = u16 0 items=["Voltage", "Current"] ("Source Mode  (0: Voltage)")
                          n426 = call "Ke2400 Configure Output.vi"("Source Mode  (0: Voltage)"=w1728, "error in (no error)"=w1713, "Compliance  Level (0.1)"=0.1, "Output Level (0)"=w1732, "VISA resource name"=w1734) -> ("error out"=w1740:errorcluster, "VISA resource name out"=w1738:refnum<visa-resource-name>)  [unwired: 5 in]
                          n427 = Number To Fractional String(number=w1732) -> (F-format string=w1731:string)  [unwired: 3 in]
                          n428 = call "Ke2400 Enable.vi"("error in (no error)"=w1740, "ON/OFF"=TRUE ("Enable Output (T: Enable)"), "VISA resource name"=w1738) -> ("error out"=w1741:errorcluster, "VISA resource name out"=w1736:refnum<visa-resource-name>)  [unwired: 7 in]
                          n429 = call "Delay.vi"("milliseconds to wait"=u32 10, "error in (no error)"=w1741) -> ("error out"=w1727:errorcluster)  [unwired: 9 in]
                          n430 = call "WS1050 AD7747 READ 36 DUT.vi"("error in"=w1727, "Log (T)"=w1711, "DUT Mask Mode (All)"=WSVCAP_SHL_I2C_DUT_Mask_Mode_Enum."C1") -> ("error out"=w1724:errorcluster, "AD7747 Values"=w1726:string[][])  [unwired: 7 in]
                          n431 = for {
                            tunnel: w1726 -> [w1752] mode=indexing
                            tunnel: [w1753] -> w1733 mode=indexing
                            tunnel: w1724 -> [w1751]
                            tunnel: [w1751] -> w1723
                            n432 = Index Array(array=w1752, index=1) -> (element=w1753:string)
                          }
                          n433 = for {
                            N: 36 -> [_]
                            tunnel: w1731 -> [w1750]
                            tunnel: [w1750] -> w1729 mode=indexing
                          }
                          n434 = call "WS1050 AD7747 READ 36 DUT.vi"("error in"=w1723, "Log (T)"=w1711, "DUT Mask Mode (All)"=WSVCAP_SHL_I2C_DUT_Mask_Mode_Enum."C2") -> ("error out"=w1721:errorcluster, "AD7747 Values"=w1719:string[][])  [unwired: 7 in]
                          n435 = for {
                            tunnel: w1719 -> [w1747] mode=indexing
                            tunnel: [w1748] -> w1720 mode=indexing
                            tunnel: w1721 -> [w1746]
                            tunnel: [w1746] -> w1718
                            n436 = Index Array(array=w1747, index=3) -> (element=w1748:string)
                          }
                          n437 = call "WS1050 AD7747 READ 36 DUT.vi"("error in"=w1718, "Log (T)"=w1711, "DUT Mask Mode (All)"=WSVCAP_SHL_I2C_DUT_Mask_Mode_Enum."C3") -> ("error out"=w1716:errorcluster, "AD7747 Values"=w1715:string[][])  [unwired: 7 in]
                          n438 = local write "STATUS"("VSA Testing...." ("STATUS")) -> ()
                          n439 = for {
                            tunnel: w1715 -> [w1743] mode=indexing
                            tunnel: [w1744] -> w1714 mode=indexing
                            tunnel: w1716 -> [w1742]
                            tunnel: [w1742] -> w1712
                            n440 = Index Array(array=w1743, index=5) -> (element=w1744:string)
                          }
                        }
                      }
                    }
                  }
                  frame True {
                    w1757 = string[][] []
                  }
                }
                n441 = Transpose 2D Array(2D array=w1656) -> (transposed array=w1654:string[][])
                n442 = Transpose 2D Array(2D array=w1655) -> (transposed array=w1653:string[][])
                n443 = Transpose 2D Array(2D array=w1652) -> (transposed array=w1651:string[][])
                n444 = Transpose 2D Array(2D array=w1649) -> (transposed array=w1648:string[][])
                n445 = call "WS1050_VSA_Convert_Data.vi"("VSA_C3"=w1648, "error in (no error)"=w1650, "VSA_C2"=w1651, "VSA_C1"=w1653, "Voltage"=w1654) -> ("error out"=w1647:errorcluster, "VSA_V3"=w1644:string[][], "VSA_V2"=w1645:string[][], "VSA_V1"=w1646:string[][])  [unwired: 3 in]
                "VSA_V1" <- w1646
                "VSA_V2" <- w1645
                "VSA_V3" <- w1644
                n446 = case shown="True" w1637 {
                  tunnel: w1666 -> [w1760 w1766]
                  tunnel: [w1760 w1765] -> w1665
                  tunnel: w1647 -> [w1759 w1764]
                  tunnel: [w1759 w1761] -> w1664
                  frame False {
                  }
                  frame True {
                    w1762 = u16 0 items=["Voltage", "Current"] ("Source Mode  (0: Voltage)")
                    n447 = call "Ke2400 Configure Output.vi"("Source Mode  (0: Voltage)"=w1762, "error in (no error)"=w1764, "Output Level (0)"=0.0, "VISA resource name"=w1766) -> ("error out"=w1761:errorcluster, "VISA resource name out"=w1765:refnum<visa-resource-name>)  [unwired: 6 in]
                  }
                }
                n448 = call "Delay.vi"("milliseconds to wait"=u32 50, "error in (no error)"=w1664) -> ("error out"=w1663:errorcluster)  [unwired: 9 in]
              }
              frame #6 {
                # "Handshake Check and EFuse Readback"
                n449 = Or(x=w1775, y=w1785) -> (x .or. y?=w1784:bool)
                n450 = Add(x=w1797, y=w1796) -> (x+y=w1783:u64)
                n451 = case shown="False" w1784 {
                  tunnel: w1810 -> [w1823 _]
                  tunnel: w1809 -> [w1822 w1828]
                  tunnel: [w1821 w1828] -> w1808
                  tunnel: w1807 -> [w1820 _]
                  tunnel: w1806 -> [w1819 _]
                  tunnel: w1805 -> [w1818 _]
                  tunnel: [w1814 w1827] -> w1804
                  tunnel: [w1813 w1827] -> w1799
                  tunnel: w1783 -> [w1812 _]
                  tunnel: w1790 -> [w1811 _]
                  frame False {
                    n452 = call "WS1050_36DUT_Handshake Check R1_Record All Regs Ver1.0.vi"("file path (use dialog)"=w1823, "Reg1_Bit Cntrl"="Reg1_Bit Cntrl", "File Name"=w1811, "SN"=w1818, "Loop"=w1812, "error"=w1822, "Lot #"=w1820, "Wafer #"=w1819) -> ("Pass/Fail"=→"EFuse Readback Status":bool[], "EFuse Read back"=w1813:string[], "Status"=w1814:string[], "error out"=w1821:errorcluster)  [unwired: 6 in, 2 out]
                    n453 = case shown="1, Default" w1812 {
                      tunnel: w1813 -> [w1824 w1825]
                      frame 0 {
                        "EFuse RB T0" <- w1824
                      }
                      frame 1, Default {
                        "Current EFuse Read back" <- w1825
                      }
                    }
                    n454 = local write "STATUS"("Hand Shake & EFuse Readback...." ("STATUS")) -> ()
                  }
                  frame True {
                    n455 = for {
                      N: 36 -> [_]
                      tunnel: [""] -> w1827 mode=indexing
                    }
                  }
                }
                n456 = Add(x=w1783, y=w1780) -> (x+y=w1781:u64)
                "TTCompleted" <- w1781
                n457 = Number To Engineering String(4:w1781) -> (0:w1795:string)  [unwired: 3 in]
                n458 = Build Array(w1794, w1792, w1791) -> (w1793:string[])
              }
              frame #7 {
                # "Save Data"
                n459 = Increment(x=w1843) -> (x+1=w1842:i32)
                n460 = Multiply(x=w1842, y=36) -> (x*y=w1837:i32)
                n461 = Path To String(path=w1847) -> (string=w1846:string)
                n462 = Bundle("Test Program"=w1878, "Comment"=w1877, "Data Out"=w1854, "Data Out"=w1853, "Data Out"=w1852, w1851, "Data Out"=w1850, "Data Out"=w1849, "Data Out"=w1848, "Freq(Hz)"=w1835, "Board#"=w1833) -> (w1834:T8)  [unwired: 1 in]
                n463 = case shown="False" w1832 {
                  tunnel: w1883 -> [w1911 w1913]
                  tunnel: [w1910 w1913] -> w1882
                  tunnel: w1881 -> [w1909 _]
                  tunnel: w1880 -> [w1908 _]
                  tunnel: w1879 -> [w1907 _]
                  tunnel: w1876 -> [w1906 _]
                  tunnel: w1874 -> [w1905 _]
                  tunnel: w1873 -> [w1904 _]
                  tunnel: w1872 -> [w1903 _]
                  tunnel: w1871 -> [w1902 _]
                  tunnel: w1870 -> [w1901 _]
                  tunnel: w1867 -> [w1900 _]
                  tunnel: w1866 -> [w1899 _]
                  tunnel: w1865 -> [w1898 _]
                  tunnel: w1863 -> [w1897 _]
                  tunnel: w1862 -> [w1896 _]
                  tunnel: w1861 -> [w1895 _]
                  tunnel: w1860 -> [w1894 _]
                  tunnel: w1859 -> [w1893 _]
                  tunnel: w1858 -> [w1892 _]
                  tunnel: w1857 -> [w1891 _]
                  tunnel: w1856 -> [w1890 _]
                  tunnel: w1855 -> [w1889 _]
                  tunnel: w1847 -> [w1888 _]
                  tunnel: w1840 -> [w1887 _]
                  tunnel: w1834 -> [w1886 _]
                  tunnel: ["Save Data...." ("STATUS") "Stop test..." ("STATUS")] -> w1831
                  tunnel: w1830 -> [w1884 _]
                  frame False {
                    n464 = call "WS1050_36 DUT SData Ver1.5a.vi"("TMN DC\\CAP Data Log File Path"=w1888, "Lot#"=w1908, "Total Delta C1(pF)"=w1891, "VSA_V1"=w1899, "Wafer#"=w1906, "File Name"=w1887, "Total Delta C2(pF)"=w1890, "error in"=w1911, "TP/Comment"=w1886, "EFuse"=w1902, "Data Output C3"=w1893, "Temperature"=w1897, "VSA_V2"=w1900, "VPI C3"=w1895, "Data Output C1"=w1905, "VPI C2"=w1894, "SN"=w1909, "R/W Status"=w1907, "Cap Header"=w1896, "HD/Cycles Completed"=w1901, "Data Output C2"=w1892, "STress Beams"=w1884, "VSA_V3"=w1898, "Current"=w1904, "VPI C1"=w1903, "Total Delta C3(pF)"=w1889) -> ("error out"=w1910:errorcluster)  [unwired: 1 in]
                  }
                  frame True {
                  }
                }
                n465 = case shown="True" "Debug" {
                  tunnel: w1837 -> [w1914 w1917]
                  tunnel: [w1914 w1915] -> w1836
                  frame False {
                  }
                  frame True {
                    n466 = Multiply(x=w1917, y="No of Rows\nFrom Spread Sheet") -> (x*y=w1915:i32)
                  }
                }
                n467 = local write "STATUS"(w1831) -> ()
                n468 = Concatenate Strings(w1846, "\\" ("string"), w1840, "_Multi Socket Data.csv" ("string")) -> (w1845:string)
              }
              frame #8 {
                n469 = case shown="True" "Plot Delta Cmin" {
                  tunnel: w1923 -> [w1937 w1952]
                  tunnel: [w1937 w1948] -> w1922
                  tunnel: w1921 -> [_ w1944]
                  tunnel: w1919 -> [_ w1942]
                  frame False {
                  }
                  frame True {
                    n470 = String To Path(string=w1944) -> (path=w1943:path)
                    n471 = call "Delay.vi"("milliseconds to wait"=u32 50, "error in (no error)"=w1952) -> ("error out"=w1951:errorcluster)  [unwired: 9 in]
                    n472 = call "36DUT Plot From Spread Sheet Ver1.5a.vi"("Plot"="Plot", "No of Rows"=w1942, "error in (no error)"=w1951, "Bank"="Bank C1", "file path (dialog if empty)"=w1943) -> ("error out"=w1946:errorcluster, "Delta C_Min Plot"=→"Min Plot_1":dbl[][])  [unwired: 5 in]
                    n473 = call "36DUT Plot From Spread Sheet Ver1.5a.vi"("Plot"="Plot", "No of Rows"=w1942, "error in (no error)"=w1946, "Bank"="Bank C2", "file path (dialog if empty)"=w1943) -> ("error out"=w1947:errorcluster, "Delta C_Min Plot"=→"Min Plot_2":dbl[][])  [unwired: 5 in]
                    n474 = call "36DUT Plot From Spread Sheet Ver1.5a.vi"("Plot"="Plot", "No of Rows"=w1942, "error in (no error)"=w1947, "Bank"="Bank C3", "file path (dialog if empty)"=w1943) -> ("error out"=w1948:errorcluster, "Delta C_Min Plot"=→"Min Plot_3":dbl[][])  [unwired: 5 in]
                  }
                }
                n475 = Get Date/Time In Seconds() -> (seconds since 1Jan1904=w1930:timestamp)
                n476 = Get Date/Time String(seconds (now)=w1930, want seconds? (F)=TRUE) -> (date string=→"date string":string, time string=→"Previous Time":string)  [unwired: 1 in]
                n477 = Greater Or Equal?(x=w1927, y="Set Stress run") -> (x >= y?=w1934:bool)
                n478 = Greater Or Equal?(x=w1926, y="TTF Completed") -> (x >= y?=w1925:bool)
                "Completed Stress" <- w1927
              }
            }
            n479 = Increment(x=w543) -> (x+1=→"Loop \ncompleted":i32)
            n480 = call "Delay.vi"("milliseconds to wait"=u32 10, "error in (no error)"=w435) -> ("error out"=w436:errorcluster)  [unwired: 9 in]
            n481 = Compound Arithmetic op=OR(w612, w513, w539) -> (w552:bool)
          }
          "Total Time" <- w372
          n482 = Increment(x=w370) -> (x+1=→"Run Loops":i32)
          n483 = local write "Completed Stress"(u64 0 ("No of HD/Cycle\nCompleted")) -> ()
          n484 = Unbundle By Name(w362) -> ("status"=w376:bool)
          n485 = Compound Arithmetic op=OR(w376, w368, w367) -> (w351:bool)
        }
        n486 = flat-sequence {
          tunnel: w283 -> [w341]
          tunnel: [w341] -> w282
          tunnel: [w340] -> w281
          tunnel: w280 -> [w340]
          frame #0 {
            n487 = One Button Dialog(message="Done!") -> ()  [unwired: 1 in, 1 out]
            n488 = local write "STATUS"("Completed!" ("STATUS")) -> ()
          }
        }
        n489 = for {
          tunnel: w304 -> [w1964]
          tunnel: w289 -> [w1963]
          tunnel: w333 -> [w1961] mode=indexing
          tunnel: [w1956] -> w303
          tunnel: [w1960] -> w332
          n490 = call "E3631A_Voltage Controller updated.vi"("VISA resource name"=w1963, "I_VDD(A)"=0.5, "Channel Controller"=w1961, "Voltage 1"=0.0, "Voltage 2"=3.3, "error in (no error)"=w1964, "I_3.3V (A)"=0.5) -> ("VISA resource name out"=w1960:refnum<visa-resource-name>, "error out"=w1957:errorcluster)  [unwired: 7 in]
          n491 = call "Delay.vi"("milliseconds to wait"=u32 100, "error in (no error)"=w1957) -> ("error out"=w1956:errorcluster)  [unwired: 9 in]
        }
        n492 = VISA Write(VISA resource name=w323, write buffer="SOUR:FUNC VOLT;VOLT:MODE FIX;RANG 100;LEV 0.0;:SENS:FUNC \"CURR\";CURR:PROT 60E-3;RANG 100E-3;:OUTP ON", error in (no error)=w304) -> (VISA resource name out=w321:refnum<visa-resource-name>, error out=w283:errorcluster)  [unwired: 1 out]
        n493 = Merge Errors(w303, w282) -> (w322:errorcluster)
      }
      frame True {
      }
    }
    n494 = Wait Until Next ms Multiple(millisecond multiple=u32 100) -> ()  [unwired: 1 out]
    n495 = Unbundle By Name(w66) -> ("status"=w65:bool)
    n496 = Compound Arithmetic op=OR(w64, w65, w86) -> (w94:bool)
    "STATUS" <- "Idle...." ("STATUS")
  }
  "Ke2000 Out" <- w10
  n497 = local write "stop During HD/Cycles"(w16) -> ()
  n498 = local write "stop"(w16) -> ()
  n499 = case shown="True" w25 {
    tunnel: [w1981 w1984] -> w8
    tunnel: w4 -> [w1981 w1983]
    frame False {
    }
    frame True {
      n500 = local write "Online"(FALSE ("Online")) -> ()
      n501 = call "WSVCAP SHL Host TL Close.vi"("error in"=w1983) -> ("error out"=w1984:errorcluster)  [unwired: 14 in]
    }
  }
  "error out" <- w8
  n502 = VISA Write(VISA resource name=w20, write buffer="SOUR:FUNC VOLT;VOLT:MODE FIX;RANG 100;LEV 0.0;:SENS:FUNC \"CURR\";CURR:PROT 60E-3;RANG 100E-3;:OUTP OFF", error in (no error)=w4) -> (VISA resource name out=→"VISA resource name out":refnum<visa-resource-name>, error out=w7:errorcluster)  [unwired: 1 out]
  n503 = VISA Write(VISA resource name=w5, write buffer=":INST:NSEL 1; :VOLT 0.000000;:OUTP 1;", error in (no error)=w4) -> (VISA resource name out=→"PS1 Out":refnum<visa-resource-name>, error out=w3:errorcluster)  [unwired: 1 out]
  n504 = Merge Errors(w3, w8, w7) -> (→"error out 2":errorcluster)
